vi "Unicorn.vi"() -> ()   [LabVIEW 2017, in "LV_Unicorn.lvlib"]
uses:
  LV_Unicorn.lvlib
  Control/AnswerUDP.ctl
  Control/unicorn_Param.ctl
  Control/unicorn_conn.ctl
  Control/unicorn_JSON.ctl
  Control/unicorn_ParamInt.ctl
  Control/unicorn_Telemetry.ctl
  Control/unicorn_Table.ctl
  Control/unicorn_ParamFloat.ctl
  Control/unicorn_array.ctl
  <vilib>/JDP Science/JSONtext/JSONtext.lvlib
panel:
  in  "FindMultiCast":bool
  in  "B_Connect":bool
  out "error out":errorcluster
  out "Ответ":string
  in  "B_Stop":bool
  in  "B_Disconnect":bool
  in  "Tab Control":T1(tab)=enum."Int"
  out "tblT":string[][](table) caption="Найденные устройства"
  in  "VersionControl":bool
  out "selDevices":T2
  in  "type_version":u32 format="%08x"
  out "devT":T2[](array[typedef])
  out "Cancel":bool
  out "ArrayUnicorn":T3
  in  "paramUnicorn":T4={"conParam"={"ReadIntParam"=TRUE, "ReadDescrParam"=FALSE, "ReadFloatParam"=TRUE, "debug"=FALSE, "ReadJSON"=TRUE, "IP_address"="192.168.1.227", "N_attempts"=5, "type_con"=enum."TCP", "MB_address"=1, "VISA"="COM1", "connection ID"=refnum, "nameDevices"="?`ОЦв-12, buld id Sep 17 2024 15:23:59", "timeout"=1000, "port"=2001, "type_version"="0A030001", "baud_rate"=115200, "VersionControl"=TRUE, "TCP_conn"=TRUE, "WindowSize"=700}, "Param"={"NumParam"={"NTelem"=201, "NInt"=16, "NFloat"=10, "NTable"=2}, "ParamInt"=[{"ID"="Режим работы", "Num"=0, "Name"="", "Type"="", "Enum"="", "Desc"="", "Unit"="", "Access"="", "FormatStr"="", "Min"=0, "Max"=0}, {"ID"="", "Num"=0, "Name"="", "Type"="", "Enum"="", "Desc"="", "Unit"="", "Access"="", "FormatStr"="", "Min"=0, "Max"=0}, {"ID"="", "Num"=0, "Name"="", "Type"="", "Enum"="", "Desc"="", "Unit"="", "Access"="", "FormatStr"="", "Min"=0, "Max"=0}, {"ID"="", "Num"=0, "Name"="", "Type"="", "Enum"="", "Desc"="", "Unit"="", "Access"="", "FormatStr"="", "Min"=0, "Max"=0}, {"ID"="", "Num"=0, "Name"="", "Type"="", "Enum"="", "Desc"="", "Unit"="", "Access"="", "FormatStr"="", "Min"=0, "Max"=0}, {"ID"="", "Num"=0, "Name"="", "Type"="", "Enum"="", "Desc"="", "Unit"="", "Access"="", "FormatStr"="", "Min"=0, "Max"=0}, {"ID"="ModeWork", "Num"=0, "Name"="", "Type"="", "Enum"="", "Desc"="", "Unit"="", "Access"="", "FormatStr"="", "Min"=0, "Max"=0}], "Telemetry"=[], "Table"=[], "ParamFloat"=[]}}
  in  "Pretty print":bool=TRUE
  out "JSONStr":string="{ \"UUID\": true, \"Reset\": false, \"Enums\": [ { \"ID\": \"Enum_LPF\", \"Name\": \"ФНЧ приемников\", \"Desc\": \"Частота среза фильтров низких частот\", \"Values\": [ { \"Name\": \"100\", \"Value\": 0, \"Desc\": \"\" }, { \"Name\": \"140\", \"Value\": 1, \"Desc\": \"\" } ] }, { \"ID\": \"Enum_HPF\", \"Name\": \"ФВЧ приемников\", \"Desc\": \"Частота среза фильтров высоких частот\", \"Values\": [ { \"Name\": \"5\", \"Value\": 0, \"Desc\": \"\" }, { \"Name\": \"10\", \"Value\": 1, \"Desc\": \"\" }, { \"Name\": \"20\", \"Value\": 2, \"Desc\": \"\" }, { \"Name\": \"40\", \"Value\": 3, \"Desc\": \"\" } ] }, { \"ID\": \"OnOffEnum\", \"Name\": \"On-off enum\", \"Num\": 0, \"Values\": [ { \"Name\": \"Выключено\", \"Value\": 0 }, { \"Name\": \"Включено\", \"Value\": 1 } ] } ], \"ParamInt\": [ { \"ID\": \"IPModeWork\", \"Num\": 0, \"Name\": \"Режим сканирования\", \"Type\": \"enum\", \"Enum\": \"OnOffEnum\", \"Desc\": \"Включение режима выполнения циклов сканирования\", \"Unit\": \"\", \"Access\": \"ro\" }, { \"ID\": \"IPStatusLF_EU\", \"Num\": 1, \"Name\": \"Состояние ЭБ НЧ\", \"Type\": \"Regular\", \"Desc\": \"Наличие ошибок в работе функциональных узлов ЭБ НЧ, при не нулевом значении светодиод «Состояние» мигает желтым или красным цветом\", \"Min\": 0, \"Max\": 0, \"Unit\": \"\", \"FormatStr\": \"0x%08x\", \"Access\": \"ro\" }, { \"ID\": \"IPGenNumber\", \"Num\": 2, \"Name\": \"Номер датчика для возбуждения\", \"Type\": \"Regular\", \"Desc\": \"Номер генератора который будет осуществлять возбуждение УЗ колебаний в ОК при помощи ПЭП, значение 0 отключает все генераторы\", \"Min\": 0, \"Max\": 16, \"Unit\": \"\", \"FormatStr\": \"%d\", \"Access\": \"rw\" }, { \"ID\": \"IPNumOfAvg\", \"Num\": 3, \"Name\": \"Количество усреднений принятых эхосигналов\", \"Type\": \"Regular\", \"Desc\": \"Количество повторений зондирования для усреднения принятых сигналов с ПЭП\", \"Min\": 1, \"Max\": 1023, \"Unit\": \"\", \"FormatStr\": \"%d\", \"Access\": \"rw\" }, { \"ID\": \"IPLPFilter\", \"Num\": 4, \"Name\": \"ФНЧ приемников\", \"Type\": \"enum\", \"Enum\": \"Enum_LPF\", \"Desc\": \"Частота среза фильтров низких частот приемников сигналов ПЭП\", \"Unit\": \"кГц\", \"Access\": \"rw\" }, { \"ID\": \"IPHPFilter\", \"Num\": 5, \"Name\": \"ФВЧ приемников\", \"Type\": \"enum\", \"Enum\": \"Enum_HPF\", \"Desc\": \"Частота среза фильтров высоких частот приемников сигналов ПЭП\", \"Unit\": \"кГц\", \"Access\": \"rw\" }, { \"ID\": \"IPModeTGC\", \"Num\": 6, \"Name\": \"Режим работы узла ВРЧ\", \"Desc\": \"Выбор режима работы узла управления временной регулировкой чувствительности\", \"Type\": \"enum\", \"Unit\": \"\", \"Access\": \"rw\", \"Enum\": { \"ID\": \"ModeTGCEnum\", \"Values\": [ { \"Desc\": \"В режиме «статический» используется не зависящая от времени чувствительность приемника\", \"Name\": \"Статический\", \"Value\": 0 }, { \"Desc\": \"В режиме «линейный» задается наклон изменения чувствительности в дБ/мс\", \"Name\": \"Линейный\", \"Value\": 1 }, { \"Desc\": \"В режиме «по таблице» значение чувствительности изменяется в соответствии с законом заданном в табличном виде\", \"Name\": \"По таблице\", \"Value\": 2 } ] } }, { \"ID\": \"IPFPGATypeVer\", \"Num\": 7, \"Name\": \"Тип и версия ПЛИС\", \"Type\": \"Regular\", \"Desc\": \"Тип и версия встроенного ПО ПЛИС платы АЦП ЭБ НЧ\", \"Unit\": \"\", \"FormatStr\": \"0x%08x\", \"Access\": \"ro\" }, { \"ID\": \"IPFPGABuildTime\", \"Num\": 8, \"Name\": \"Дата сборки ПО ПЛИС\", \"Type\": \"Regular\", \"Desc\": \"Дата сборки встроенного ПО ПЛИС платы АЦП\", \"Unit\": \"UNIX Time\", \"FormatStr\": \"%d\", \"Access\": \"ro\" }, { \"ID\": \"IPADCMonMCUBuildTime\", \"Num\": 9, \"Name\": \"Дата сборки ПО МК мониторинга платы АЦП\", \"Type\": \"Regular\", \"Desc\": \"Дата сборки ПО МК мониторинга платы АЦП\", \"Unit\": \"UNIX Time\", \"FormatStr\": \"%d\", \"Access\": \"ro\" }, { \"ID\": \"IPPMD2MCUBuildTime\", \"Num\": 10, \"Name\": \"Дата сборки ПО МК мониторинга ИП D2\", \"Type\": \"Regular\", \"Desc\": \"Дата сборки ПО МК мониторинга платы источника питания D2\", \"Unit\": \"UNIX Time\", \"FormatStr\": \"%d\", \"Access\": \"ro\" }, { \"ID\": \"IPPMD4MCUBuildTime\", \"Num\": 11, \"Name\": \"Дата сборки ПО МК мониторинга ИП D6\", \"Type\": \"Regular\", \"Desc\": \"Дата сборки ПО МК мониторинга платы источника питания D6\", \"Unit\": \"UNIX Time\", \"FormatStr\": \"%d\", \"Access\": \"ro\" }, { \"ID\": \"IPDefaultAddress\", \"Num\": 12, \"Name\": \"IP адрес электронного блока по умолчанию\", \"Type\": \"IPv4Addr\", \"Desc\": \"Присваивается электронному блоку если не был получен автоматически от DCHP сервера\", \"Unit\": \"IPv4\", \"Access\": \"rw\" }, { \"ID\": \"IPDefaultNetMask\", \"Num\": 13, \"Name\": \"Маска подсети\", \"Type\": \"IPv4Mask\", \"Desc\": \"Присваивается электронному блоку если не был получен автоматически от DCHP сервера\", \"Unit\": \"IPv4\", \"Access\": \"rw\" }, { \"ID\": \"IPDefaultGW\", \"Num\": 14, \"Name\": \"Основной шлюз \", \"Type\": \"IPv4Addr\", \"Desc\": \"Присваивается электронному блоку если не был получен автоматически от DCHP сервера\", \"Unit\": \"IPv4\", \"Access\": \"rw\" }, { \"ID\": \"IPSaveParem\", \"Num\": 15, \"Name\": \"Сохранение параметров\", \"Type\": \"bool\", \"Desc\": \"Сохранение параметров в энергонезависимую память\", \"Unit\": \"\", \"FormatStr\": \"\", \"Access\": \"rw\" } ], \"ParamFloat\": [ { \"ID\": \"FPFreqRepExPulses\", \"Num\": 0, \"Name\": \"Частота повторения импульсов возбуждения\", \"Desc\": \"Максимальная частота с которой будут формироваться импульсы возбуждения ПЭП\", \"Type\": \"Regular\", \"Unit\": \"Гц\", \"FormatStr\": \"%.1f\", \"Min\": 1.0, \"Max\": 20.0, \"Access\": \"rw\" }, { \"ID\": \"FPFreqExFilling\", \"Num\": 1, \"Name\": \"Частота сигнала заполнения импульса возбуждения\", \"Desc\": \"Частота сигнала заполнения импульса возбуждения ПЭП\", \"Type\": \"Regular\", \"Unit\": \"кГц\", \"FormatStr\": \"%.1f\", \"Min\": 10.0, \"Max\": 100.0, \"Access\": \"rw\" }, { \"ID\": \"FPNumPerFillExPulse\", \"Num\": 2, \"Name\": \"Количество периодов заполнения импульса возбуждения\", \"Desc\": \"Количество периодов частоты сигнала заполнения в импульсе возбуждения ПЭП\", \"Type\": \"Regular\", \"Unit\": \"шт\", \"FormatStr\": \"%.1f\", \"Min\": 1.0, \"Max\": 10.0, \"Access\": \"rw\" }, { \"ID\": \"FPAmplExPulse\", \"Num\": 3, \"Name\": \"Амплитуда импульса возбуждения\", \"Desc\": \"Максимальная амплитуда импульса возбуждения ПЭП, 100 % соответствуют 150 В амплитуды или 300 В размаха сигнала возбуждения ПЭП\", \"Type\": \"Regular\", \"Unit\": \"%\", \"FormatStr\": \"%.1f\", \"Min\": 0.0, \"Max\": 100.0, \"Access\": \"rw\" }, { \"ID\": \"FPDelayExPulse\", \"Num\": 4, \"Name\": \"Задержка начала импульса возбуждения\", \"Desc\": \"Задержка начала импульса возбуждения относительно импульса синхронизации\", \"Type\": \"Regular\", \"Unit\": \"мкс\", \"FormatStr\": \"%.2f\", \"Min\": 0.0, \"Max\": 50.0, \"Access\": \"rw\" }, { \"ID\": \"FPScanAreaDelay\", \"Num\": 5, \"Name\": \"Задержка области сканирования\", \"Desc\": \"Задержка начала области сканирования относительно импульса синхронизации, задержка начала работы приемников сигналов ПЭП\", \"Type\": \"Regular\", \"Unit\": \"мкс\", \"FormatStr\": \"%.2f\", \"Min\": 0.0, \"Max\": 100.0e3, \"Access\": \"rw\" }, { \"ID\": \"FPDurationScanArea\", \"Num\": 6, \"Name\": \"Длительность области сканирования\", \"Desc\": \"Длительность области сканирования, длительность работы приемников сигналов ПЭП\", \"Type\": \"Regular\", \"Unit\": \"мкс\", \"FormatStr\": \"%.2f\", \"Min\": 100.0, \"Max\": 15728.0, \"Access\": \"rw\" }, { \"ID\": \"FPSamplingFreq\", \"Num\": 7, \"Name\": \"Частота дискретизации сигнала принимаемого с ПЭП сигнала\", \"Desc\": \"Частота следования отсчетов амплитуды принятого с ПЭП эхосигнала\", \"Type\": \"Regular\", \"Unit\": \"Гц\", \"FormatStr\": \"%.2f\", \"Access\": \"ro\" }, { \"ID\": \"FPInitialGain\", \"Num\": 8, \"Name\": \"Начальное значение коэффициента усиления приемников\", \"Desc\": \"Значение усиления для режима работы ВРЧ «статический», для режимов «линейный» и «по таблице» используется как начальное значение усиления\", \"Type\": \"Regular\", \"Unit\": \"дБ\", \"FormatStr\": \"%.1f\", \"Min\": 0.0, \"Max\": 40.0, \"Access\": \"rw\" }, { \"ID\": \"FPRateChangeGain\", \"Num\": 9, \"Name\": \"Скорость изменения чувствительности\", \"Desc\": \"Значение скорости изменения усиления для режима работы ВРЧ «линейный», в режимах «статический» и «по таблице» не влияет на работу узла ВРЧ\", \"Type\": \"Regular\", \"Unit\": \"дБ/мс\", \"FormatStr\": \"%.2f\", \"Min\": -40.0, \"Max\": 40.0, \"Access\": \"rw\" } ], \"Telemetry\": [ { \"ID\": \"CoreUptime\", \"Num\": 0, \"Name\": \"Core uptime\", \"Desc\": \"\", \"Unit\": \"s\", \"FormatStr\": \"%.1f\" }, { \"ID\": \"LCUptime\", \"Num\": 1, \"Name\": \"FPGA uptime\", \"Desc\": \"\", \"Unit\": \"s\", \"FormatStr\": \"%.1f\" }, { \"ID\": \"TelStatusLF_EU\", \"Num\": 2, \"Name\": \"TelStatusLF_EU\", \"Desc\": \"\", \"Unit\": \"\", \"Min\": -0.01, \"Max\": 0.01, \"FormatStr\": \"%.0f\" }, { \"ID\": \"TelMBVrefMin\", \"Num\": 3, \"Name\": \"TelMBVrefMin\", \"Desc\": \"\", \"Unit\": \"В\", \"Min\": 1.18, \"Max\": 1.22, \"FormatStr\": \"%.3f\" }, { \"ID\": \"TelMBVrefAvg\", \"Num\": 4, \"Name\": \"TelMBVrefAvg\", \"Desc\": \"\", \"Unit\": \"В\", \"Min\": 1.18, \"Max\": 1.22, \"FormatStr\": \"%.3f\" }, { \"ID\": \"TelMBVrefMax\", \"Num\": 5, \"Name\": \"TelMBVrefMax\", \"Desc\": \"\", \"Unit\": \"В\", \"Min\": 1.18, \"Max\": 1.22, \"FormatStr\": \"%.3f\" }, { \"ID\": \"TelMB3_3VMin\", \"Num\": 6, \"Name\": \"TelMB3_3VMin\", \"Desc\": \"\", \"Unit\": \"В\", \"Min\": 3.2, \"Max\": 3.45, \"FormatStr\": \"%.3f\" }, { \"ID\": \"TelMB3_3VAvg\", \"Num\": 7, \"Name\": \"TelMB3_3VAvg\", \"Desc\": \"\", \"Unit\": \"В\", \"Min\": 3.2, \"Max\": 3.45, \"FormatStr\": \"%.3f\" }, { \"ID\": \"TelMB3_3VMax\", \"Num\": 8, \"Name\": \"TelMB3_3VMax\", \"Desc\": \"\", \"Unit\": \"В\", \"Min\": 3.2, \"Max\": 3.45, \"FormatStr\": \"%.3f\" }, { \"ID\": \"TelMB3_3VcMin\", \"Num\": 9, \"Name\": \"TelMB3_3VcMin\", \"Desc\": \"\", \"Unit\": \"В\", \"Min\": 3.2, \"Max\": 3.45, \"FormatStr\": \"%.3f\" }, { \"ID\": \"TelMB3_3VcAvg\", \"Num\": 10, \"Name\": \"TelMB3_3VcAvg\", \"Desc\": \"\", \"Unit\": \"В\", \"Min\": 3.2, \"Max\": 3.45, \"FormatStr\": \"%.3f\" }, { \"ID\": \"TelMB3_3VcMax\", \"Num\": 11, \"Name\": \"TelMB3_3VcMax\", \"Desc\": \"\", \"Unit\": \"В\", \"Min\": 3.2, \"Max\": 3.45, \"FormatStr\": \"%.3f\" }, { \"ID\": \"TelMB1_8VcMin\", \"Num\": 12, \"Name\": \"TelMB1_8VcMin\", \"Desc\": \"\", \"Unit\": \"В\", \"Min\": 1.65, \"Max\": 1.95, \"FormatStr\": \"%.3f\" }, { \"ID\": \"TelMB1_8VcAvg\", \"Num\": 13, \"Name\": \"TelMB1_8VcAvg\", \"Desc\": \"\", \"Unit\": \"В\", \"Min\": 1.65, \"Max\": 1.95, \"FormatStr\": \"%.3f\" }, { \"ID\": \"TelMB1_8VcMax\", \"Num\": 14, \"Name\": \"TelMB1_8VcMax\", \"Desc\": \"\", \"Unit\": \"В\", \"Min\": 1.65, \"Max\": 1.95, \"FormatStr\": \"%.3f\" }, { \"ID\": \"TelMB5VcMin\", \"Num\": 15, \"Name\": \"TelMB5VcMin\", \"Desc\": \"\", \"Unit\": \"В\", \"Min\": 4.8, \"Max\": 5.25, \"FormatStr\": \"%.3f\" }, { \"ID\": \"TelMB5VcAvg\", \"Num\": 16, \"Name\": \"TelMB5VcAvg\", \"Desc\": \"\", \"Unit\": \"В\", \"Min\": 4.8, \"Max\": 5.25, \"FormatStr\": \"%.3f\" }, { \"ID\": \"TelMB5VcMax\", \"Num\": 17, \"Name\": \"TelMB5VcMax\", \"Desc\": \"\", \"Unit\": \"В\", \"Min\": 4.8, \"Max\": 5.25, \"FormatStr\": \"%.3f\" }, { \"ID\": \"TelMB5VconMin\", \"Num\": 18, \"Name\": \"TelMB5VconMin\", \"Desc\": \"\", \"Unit\": \"В\", \"Min\": 4.8, \"Max\": 5.25, \"FormatStr\": \"%.3f\" }, { \"ID\": \"TelMB5VconAvg\", \"Num\": 19, \"Name\": \"TelMB5VconAvg\", \"Desc\": \"\", \"Unit\": \"В\", \"Min\": 4.8, \"Max\": 5.25, \"FormatStr\": \"%.3f\" }, { \"ID\": \"_TelMB5VconMax\", \"Num\": 20, \"Name\": \"_TelMB5VconMax\", \"Desc\": \"\", \"Unit\": \"В\", \"Min\": 4.8, \"Max\": 5.25, \"FormatStr\": \"%.3f\" }, { \"ID\": \"TelMBTemp\", \"Num\": 21, \"Name\": \"TelMBTemp\", \"Desc\": \"\", \"Unit\": \"°C\", \"Min\": 10.0, \"Max\": 80.0, \"FormatStr\": \"%.1f\" }, { \"ID\": \"TelADCGDUptime\", \"Num\": 22, \"Name\": \"TelADCGDUptime\", \"Desc\": \"\", \"Unit\": \"s\", \"FormatStr\": \"%.0f\" }, { \"ID\": \"TelADCVRefIntMin\", \"Num\": 23, \"Name\": \"TelADCVRefIntMin\", \"Desc\": \"\", \"Unit\": \"V\", \"Min\": 1.18, \"Max\": 1.22, \"FormatStr\": \"%.3f\" }, { \"ID\": \"TelADCVRefIntAVG\", \"Num\": 24, \"Name\": \"TelADCVRefIntAVG\", \"Desc\": \"\", \"Unit\": \"V\", \"Min\": 1.18, \"Max\": 1.22, \"FormatStr\": \"%.3f\" }, { \"ID\": \"TelADCVRefIntMax\", \"Num\": 25, \"Name\": \"TelADCVRefIntMax\", \"Desc\": \"\", \"Unit\": \"V\", \"Min\": 1.18, \"Max\": 1.22, \"FormatStr\": \"%.3f\" }, { \"ID\": \"TelADCVp1_2VdMin\", \"Num\": 26, \"Name\": \"TelADCVp1_2VdMin\", \"Desc\": \"\", \"Unit\": \"V\", \"Min\": 1.18, \"Max\": 1.28, \"FormatStr\": \"%.3f\" }, { \"ID\": \"TelADCVp1_2VdAVG\", \"Num\": 27, \"Name\": \"TelADCVp1_2VdAVG\", \"Desc\": \"\", \"Unit\": \"V\", \"Min\": 1.18, \"Max\": 1.28, \"FormatStr\": \"%.3f\" }, { \"ID\": \"TelADCVp1_2VdMax\", \"Num\": 28, \"Name\": \"TelADCVp1_2VdMax\", \"Desc\": \"\", \"Unit\": \"V\", \"Min\": 1.18, \"Max\": 1.28, \"FormatStr\": \"%.3f\" }, { \"ID\": \"TelADCVp1_8VaMin\", \"Num\": 29, \"Name\": \"TelADCVp1_8VaMin\", \"Desc\": \"\", \"Unit\": \"V\", \"Min\": 1.65, \"Max\": 1.95, \"FormatStr\": \"%.3f\" }, { \"ID\": \"TelADCVp1_8VaAVG\", \"Num\": 30, \"Name\": \"TelADCVp1_8VaAVG\", \"Desc\": \"\", \"Unit\": \"V\", \"Min\": 1.65, \"Max\": 1.95, \"FormatStr\": \"%.3f\" }, { \"ID\": \"TelADCVp1_8VaMax\", \"Num\": 31, \"Name\": \"TelADCVp1_8VaMax\", \"Desc\": \"\", \"Unit\": \"V\", \"Min\": 1.65, \"Max\": 1.95, \"FormatStr\": \"%.3f\" }, { \"ID\": \"TelADCVp3_3VMin\", \"Num\": 32, \"Name\": \"TelADCVp3_3VMin\", \"Desc\": \"\", \"Unit\": \"V\", \"Min\": 3.2, \"Max\": 3.45, \"FormatStr\": \"%.3f\" }, { \"ID\": \"TelADCVp3_3VAVG\", \"Num\": 33, \"Name\": \"TelADCVp3_3VAVG\", \"Desc\": \"\", \"Unit\": \"V\", \"Min\": 3.2, \"Max\": 3.45, \"FormatStr\": \"%.3f\" }, { \"ID\": \"TelADCVp3_3VMax\", \"Num\": 34, \"Name\": \"TelADCVp3_3VMax\", \"Desc\": \"\", \"Unit\": \"V\", \"Min\": 3.2, \"Max\": 3.45, \"FormatStr\": \"%.3f\" }, { \"ID\": \"TelADCVp5VMin\", \"Num\": 35, \"Name\": \"TelADCVp5VMin\", \"Desc\": \"\", \"Unit\": \"V\", \"Min\": 4.8, \"Max\": 5.25, \"FormatStr\": \"%.3f\" }, { \"ID\": \"TelADCVp5VAVG\", \"Num\": 36, \"Name\": \"TelADCVp5VAVG\", \"Desc\": \"\", \"Unit\": \"V\", \"Min\": 4.8, \"Max\": 5.25, \"FormatStr\": \"%.3f\" }, { \"ID\": \"TelADCVp5VMax\", \"Num\": 37, \"Name\": \"TelADCVp5VMax\", \"Desc\": \"\", \"Unit\": \"V\", \"Min\": 4.8, \"Max\": 5.25, \"FormatStr\": \"%.3f\" }, { \"ID\": \"TelADCVp5VsMin\", \"Num\": 38, \"Name\": \"TelADCVp5VsMin\", \"Desc\": \"\", \"Unit\": \"V\", \"Min\": 4.8, \"Max\": 5.25, \"FormatStr\": \"%.3f\" }, { \"ID\": \"TelADCVp5VsAVG\", \"Num\": 39, \"Name\": \"TelADCVp5VsAVG\", \"Desc\": \"\", \"Unit\": \"V\", \"Min\": 4.8, \"Max\": 5.25, \"FormatStr\": \"%.3f\" }, { \"ID\": \"TelADCVp5VsMax\", \"Num\": 40, \"Name\": \"TelADCVp5VsMax\", \"Desc\": \"\", \"Unit\": \"V\", \"Min\": 4.8, \"Max\": 5.25, \"FormatStr\": \"%.3f\" }, { \"ID\": \"TelADCVp15VMin\", \"Num\": 41, \"Name\": \"TelADCVp15VMin\", \"Desc\": \"\", \"Unit\": \"V\", \"Min\": 14.5, \"Max\": 15.5, \"FormatStr\": \"%.3f\" }, { \"ID\": \"TelADCVp15VAVG\", \"Num\": 42, \"Name\": \"TelADCVp15VAVG\", \"Desc\": \"\", \"Unit\": \"V\", \"Min\": 14.5, \"Max\": 15.5, \"FormatStr\": \"%.3f\" }, { \"ID\": \"TelADCVp15VMax\", \"Num\": 43, \"Name\": \"TelADCVp15VMax\", \"Desc\": \"\", \"Unit\": \"V\", \"Min\": 14.5, \"Max\": 15.5, \"FormatStr\": \"%.3f\" }, { \"ID\": \"TelADCVn5VMin\", \"Num\": 44, \"Name\": \"TelADCVn5VMin\", \"Desc\": \"\", \"Unit\": \"V\", \"Min\": -5.25, \"Max\": -4.8, \"FormatStr\": \"%.3f\" }, { \"ID\": \"TelADCVn5VAVG\", \"Num\": 45, \"Name\": \"TelADCVn5VAVG\", \"Desc\": \"\", \"Unit\": \"V\", \"Min\": -5.25, \"Max\": -4.8, \"FormatStr\": \"%.3f\" }, { \"ID\": \"TelADCVn5VMax\", \"Num\": 46, \"Name\": \"TelADCVn5VMax\", \"Desc\": \"\", \"Unit\": \"V\", \"Min\": -5.25, \"Max\": -4.8, \"FormatStr\": \"%.3f\" }, { \"ID\": \"TelADCVn15VMin\", \"Num\": 47, \"Name\": \"TelADCVn15VMin\", \"Desc\": \"\", \"Unit\": \"V\", \"Min\": -15.5, \"Max\": -14.5, \"FormatStr\": \"%.3f\" }, { \"ID\": \"TelADCVn15VAVG\", \"Num\": 48, \"Name\": \"TelADCVn15VAVG\", \"Desc\": \"\", \"Unit\": \"V\", \"Min\": -15.5, \"Max\": -14.5, \"FormatStr\": \"%.3f\" }, { \"ID\": \"TelADCVn15VMax\", \"Num\": 49, \"Name\": \"TelADCVn15VMax\", \"Desc\": \"\", \"Unit\": \"V\", \"Min\": -15.5, \"Max\": -14.5, \"FormatStr\": \"%.3f\" }, { \"ID\": \"TelADCTempSensor\", \"Num\": 50, \"Name\": \"TelADCTempSensor\", \"Desc\": \"\", \"Unit\": \"°C\", \"Min\": 10.0, \"Max\": 80.0, \"FormatStr\": \"%.1f\" }, { \"ID\": \"TelGD32E230PassPacketCount\", \"Num\": 51, \"Name\": \"TelGD32E230PassPacketCount\", \"Desc\": \"\", \"Unit\": \"\", \"FormatStr\": \"%.0f\" }, { \"ID\": \"TelGD32E230ErrorPacketCount\", \"Num\": 52, \"Name\": \"TelGD32E230ErrorPacketCount\", \"Desc\": \"\", \"Unit\": \"\", \"FormatStr\": \"%.0f\" }, { \"ID\": \"TelPMD2Up_time\", \"Num\": 53, \"Name\": \"PM D2 Uptime\", \"Desc\": \"\", \"Unit\": \"s\", \"FormatStr\": \"%.0f\" }, { \"ID\": \"TelPMD2CInMin\", \"Num\": 54, \"Name\": \"TelPMD2CInMin\", \"Desc\": \"\", \"Unit\": \"A\", \"Min\": 0.1, \"Max\": 3.15, \"FormatStr\": \"%.3f\" }, { \"ID\": \"TelPMD2CInAVG\", \"Num\": 55, \"Name\": \"TelPMD2CInAVG\", \"Desc\": \"\", \"Unit\": \"A\", \"Min\": 0.1, \"Max\": 3.15, \"FormatStr\": \"%.3f\" }, { \"ID\": \"TelPMD2CInMax\", \"Num\": 56, \"Name\": \"TelPMD2CInMax\", \"Desc\": \"\", \"Unit\": \"A\", \"Min\": 0.1, \"Max\": 3.15, \"FormatStr\": \"%.3f\" }, { \"ID\": \"TelPMD2VInMin\", \"Num\": 57, \"Name\": \"TelPMD2VInMin\", \"Desc\": \"\", \"Unit\": \"V\", \"Min\": 10.5, \"Max\": 14.0, \"FormatStr\": \"%.3f\" }, { \"ID\": \"TelPMD2VInAVG\", \"Num\": 58, \"Name\": \"TelPMD2VInAVG\", \"Desc\": \"\", \"Unit\": \"V\", \"Min\": 10.5, \"Max\": 14.0, \"FormatStr\": \"%.3f\" }, { \"ID\": \"TelPMD2VInMax\", \"Num\": 59, \"Name\": \"TelPMD2VInMax\", \"Desc\": \"\", \"Unit\": \"V\", \"Min\": 10.5, \"Max\": 14.0, \"FormatStr\": \"%.3f\" }, { \"ID\": \"TelPMD2PInMin\", \"Num\": 60, \"Name\": \"TelPMD2PInMin\", \"Desc\": \"\", \"Unit\": \"W\", \"Min\": 1.0, \"Max\": 30.0, \"FormatStr\": \"%.3f\" }, { \"ID\": \"TelPMD2PInAVG\", \"Num\": 61, \"Name\": \"TelPMD2PInAVG\", \"Desc\": \"\", \"Unit\": \"W\", \"Min\": 1.0, \"Max\": 30.0, \"FormatStr\": \"%.3f\" }, { \"ID\": \"TelPMD2PInMax\", \"Num\": 62, \"Name\": \"TelPMD2PInMax\", \"Desc\": \"\", \"Unit\": \"W\", \"Min\": 1.0, \"Max\": 30.0, \"FormatStr\": \"%.3f\" }, { \"ID\": \"TelPMD2VRefIntMin\", \"Num\": 63, \"Name\": \"TelPMD2VRefIntMin\", \"Desc\": \"\", \"Unit\": \"V\", \"Min\": 1.18, \"Max\": 1.22, \"FormatStr\": \"%.3f\" }, { \"ID\": \"TelPMD2VRefIntAVG\", \"Num\": 64, \"Name\": \"TelPMD2VRefIntAVG\", \"Desc\": \"\", \"Unit\": \"V\", \"Min\": 1.18, \"Max\": 1.22, \"FormatStr\": \"%.3f\" }, { \"ID\": \"TelPMD2VRefIntMax\", \"Num\": 65, \"Name\": \"TelPMD2VRefIntMax\", \"Desc\": \"\", \"Unit\": \"V\", \"Min\": 1.18, \"Max\": 1.22, \"FormatStr\": \"%.3f\" }, { \"ID\": \"TelPMD2ConvFreq\", \"Num\": 66, \"Name\": \"TelPMD2ConvFreq\", \"Desc\": \"\", \"Unit\": \"Hz\", \"Min\": 120.0e3, \"Max\": 135.0e3, \"FormatStr\": \"%.0f\" }, { \"ID\": \"TelPMD2TempSensor\", \"Num\": 67, \"Name\": \"TelPMD2TempSensor\", \"Desc\": \"\", \"Unit\": \"°C\", \"Min\": 10.0, \"Max\": 80.0, \"FormatStr\": \"%.1f\" }, { \"ID\": \"TelPMD6Up_time\", \"Num\": 68, \"Name\": \"PM D6 Uptime\", \"Desc\": \"\", \"Unit\": \"s\", \"FormatStr\": \"%.0f\" }, { \"ID\": \"TelPMD6Vp45VMin\", \"Num\": 69, \"Name\": \"TelPMD6Vp45VMin\", \"Desc\": \"\", \"Unit\": \"V\", \"Min\": 42.0, \"Max\": 47.0, \"FormatStr\": \"%.3f\" }, { \"ID\": \"TelPMD6Vp45VAVG\", \"Num\": 70, \"Name\": \"TelPMD6Vp45VAVG\", \"Desc\": \"\", \"Unit\": \"V\", \"Min\": 42.0, \"Max\": 47.0, \"FormatStr\": \"%.3f\" }, { \"ID\": \"TelPMD6Vp45VMax\", \"Num\": 71, \"Name\": \"TelPMD6Vp45VMax\", \"Desc\": \"\", \"Unit\": \"V\", \"Min\": 42.0, \"Max\": 47.0, \"FormatStr\": \"%.3f\" }, { \"ID\": \"TelPMD6Vn45VMin\", \"Num\": 72, \"Name\": \"TelPMD6Vn45VMin\", \"Desc\": \"\", \"Unit\": \"V\", \"Min\": -47.0, \"Max\": -42.0, \"FormatStr\": \"%.3f\" }, { \"ID\": \"TelPMD6Vn45VAVG\", \"Num\": 73, \"Name\": \"TelPMD6Vn45VAVG\", \"Desc\": \"\", \"Unit\": \"V\", \"Min\": -47.0, \"Max\": -42.0, \"FormatStr\": \"%.3f\" }, { \"ID\": \"TelPMD6Vn45VMax\", \"Num\": 74, \"Name\": \"TelPMD6Vn45VMax\", \"Desc\": \"\", \"Unit\": \"V\", \"Min\": -47.0, \"Max\": -42.0, \"FormatStr\": \"%.3f\" }, { \"ID\": \"TelPMD6Vp8VMin\", \"Num\": 75, \"Name\": \"TelPMD6Vp8VMin\", \"Desc\": \"\", \"Unit\": \"V\", \"Min\": 7.0, \"Max\": 9.5, \"FormatStr\": \"%.3f\" }, { \"ID\": \"TelPMD6Vp8VAVG\", \"Num\": 76, \"Name\": \"TelPMD6Vp8VAVG\", \"Desc\": \"\", \"Unit\": \"V\", \"Min\": 7.0, \"Max\": 9.5, \"FormatStr\": \"%.3f\" }, { \"ID\": \"TelPMD6Vp8VMax\", \"Num\": 77, \"Name\": \"TelPMD6Vp8VMax\", \"Desc\": \"\", \"Unit\": \"V\", \"Min\": 7.0, \"Max\": 9.5, \"FormatStr\": \"%.3f\" }, { \"ID\": \"TelPMD6Vp5VMin\", \"Num\": 78, \"Name\": \"TelPMD6Vp5VMin\", \"Desc\": \"\", \"Unit\": \"V\", \"Min\": 4.8, \"Max\": 5.3, \"FormatStr\": \"%.3f\" }, { \"ID\": \"TelPMD6Vp5VAVG\", \"Num\": 79, \"Name\": \"TelPMD6Vp5VAVG\", \"Desc\": \"\", \"Unit\": \"V\", \"Min\": 4.8, \"Max\": 5.3, \"FormatStr\": \"%.3f\" }, { \"ID\": \"TelPMD6Vp5VMax\", \"Num\": 80, \"Name\": \"TelPMD6Vp5VMax\", \"Desc\": \"\", \"Unit\": \"V\", \"Min\": 4.8, \"Max\": 5.3, \"FormatStr\": \"%.3f\" }, { \"ID\": \"TelPMD6Vp20VMin\", \"Num\": 81, \"Name\": \"TelPMD6Vp20VMin\", \"Desc\": \"\", \"Unit\": \"V\", \"Min\": 17.0, \"Max\": 19.0, \"FormatStr\": \"%.3f\" }, { \"ID\": \"TelPMD6Vp20VAVG\", \"Num\": 82, \"Name\": \"TelPMD6Vp20VAVG\", \"Desc\": \"\", \"Unit\": \"V\", \"Min\": 17.0, \"Max\": 19.0, \"FormatStr\": \"%.3f\" }, { \"ID\": \"TelPMD6Vp20VMax\", \"Num\": 83, \"Name\": \"TelPMD6Vp20VMax\", \"Desc\": \"\", \"Unit\": \"V\", \"Min\": 17.0, \"Max\": 19.0, \"FormatStr\": \"%.3f\" }, { \"ID\": \"TelPMD6Vn8VMin\", \"Num\": 84, \"Name\": \"TelPMD6Vn8VMin\", \"Desc\": \"\", \"Unit\": \"V\", \"Min\": -9.5, \"Max\": -7.0, \"FormatStr\": \"%.3f\" }, { \"ID\": \"TelPMD6Vn8VAVG\", \"Num\": 85, \"Name\": \"TelPMD6Vn8VAVG\", \"Desc\": \"\", \"Unit\": \"V\", \"Min\": -9.5, \"Max\": -7.0, \"FormatStr\": \"%.3f\" }, { \"ID\": \"TelPMD6Vn8VMax\", \"Num\": 86, \"Name\": \"TelPMD6Vn8VMax\", \"Desc\": \"\", \"Unit\": \"V\", \"Min\": -9.5, \"Max\": -7.0, \"FormatStr\": \"%.3f\" }, { \"ID\": \"TelPMD6Vn20VMin\", \"Num\": 87, \"Name\": \"TelPMD6Vn20VMin\", \"Desc\": \"\", \"Unit\": \"V\", \"Min\": -19.0, \"Max\": -17.0, \"FormatStr\": \"%.3f\" }, { \"ID\": \"TelPMD6Vn20VAVG\", \"Num\": 88, \"Name\": \"TelPMD6Vn20VAVG\", \"Desc\": \"\", \"Unit\": \"V\", \"Min\": -19.0, \"Max\": -17.0, \"FormatStr\": \"%.3f\" }, { \"ID\": \"TelPMD6Vn20VMax\", \"Num\": 89, \"Name\": \"TelPMD6Vn20VMax\", \"Desc\": \"\", \"Unit\": \"V\", \"Min\": -19.0, \"Max\": -17.0, \"FormatStr\": \"%.3f\" }, { \"ID\": \"TelPMD6VRefIntMin\", \"Num\": 90, \"Name\": \"TelPMD6VRefIntMin\", \"Desc\": \"\", \"Unit\": \"V\", \"Min\": 1.18, \"Max\": 1.22, \"FormatStr\": \"%.3f\" }, { \"ID\": \"TelPMD6VRefIntAVG\", \"Num\": 91, \"Name\": \"TelPMD6VRefIntAVG\", \"Desc\": \"\", \"Unit\": \"V\", \"Min\": 1.18, \"Max\": 1.22, \"FormatStr\": \"%.3f\" }, { \"ID\": \"TelPMD6VRefIntMax\", \"Num\": 92, \"Name\": \"TelPMD6VRefIntMax\", \"Desc\": \"\", \"Unit\": \"V\", \"Min\": 1.18, \"Max\": 1.22, \"FormatStr\": \"%.3f\" }, { \"ID\": \"TelPMD6TempSensor\", \"Num\": 93, \"Name\": \"TelPMD6TempSensor\", \"Desc\": \"\", \"Unit\": \"°C\", \"Min\": 10.0, \"Max\": 80.0, \"FormatStr\": \"%.1f\" }, { \"ID\": \"TelPMPassPacketCount\", \"Num\": 94, \"Name\": \"TelPMPassPacketCount\", \"Desc\": \"\", \"Unit\": \"\", \"FormatStr\": \"%.0f\" }, { \"ID\": \"TelPMErrorPacketCount\", \"Num\": 95, \"Name\": \"TelPMErrorPacketCount\", \"Desc\": \"\", \"Unit\": \"\", \"FormatStr\": \"%.0f\" } ], \"Table\": [ { \"Num\": 0, \"Access\": \"ro\", \"ColumnCount\": 18, \"DataType\": \"float\", \"FormatStr\": \"%f\", \"ID\": \"RAWADCData\", \"Name\": \"Данные АЦП\", \"NeedParamPrepare\": true, \"RowCount\": 1, \"Columns\": [ { \"Column\": 0, \"Name\": \"Ось времени\", \"Type\": \"Regular\" },{ \"Column\": 1, \"Name\": \"Датчик 1\", \"Type\": \"Regular\" },{ \"Column\": 2, \"Name\": \"Датчик 2\", \"Type\": \"Regular\" },{ \"Column\": 3, \"Name\": \"Датчик 3\", \"Type\": \"Regular\" },{ \"Column\": 4, \"Name\": \"Датчик 4\", \"Type\": \"Regular\" },{ \"Column\": 5, \"Name\": \"Датчик 5\", \"Type\": \"Regular\" },{ \"Column\": 6, \"Name\": \"Датчик 6\", \"Type\": \"Regular\" },{ \"Column\": 7, \"Name\": \"Датчик 7\", \"Type\": \"Regular\" },{ \"Column\": 8, \"Name\": \"Датчик 8\", \"Type\": \"Regular\" },{ \"Column\": 9, \"Name\": \"Датчик 9\", \"Type\": \"Regular\" },{ \"Column\": 10, \"Name\": \"Датчик 10\", \"Type\": \"Regular\" },{ \"Column\": 11, \"Name\": \"Датчик 11\", \"Type\": \"Regular\" },{ \"Column\": 12, \"Name\": \"Датчик 12\", \"Type\": \"Regular\" },{ \"Column\": 13, \"Name\": \"Датчик 13\", \"Type\": \"Regular\" },{ \"Column\": 14, \"Name\": \"Датчик 14\", \"Type\": \"Regular\" },{ \"Column\": 15, \"Name\": \"Датчик 15\", \"Type\": \"Regular\" },{ \"Column\": 16, \"Name\": \"Датчик 16\", \"Type\": \"Regular\" },{ \"Column\": 17, \"Name\": \"Коэфф. усиления\", \"Type\": \"Regular\" } ] }, { \"Num\": 1, \"ID\": \"CalibrADC\", \"Access\": \"rw\", \"ColumnCount\": 2, \"RowCount\": 16, \"DataType\": \"float\", \"FormatStr\": \"%f\", \"Name\": \"Параметры калибровки\", \"Desc\": \"Параметры калибровки каналов приема\", \"NeedParamPrepare\": false, \"Columns\": [ { \"Column\": 0, \"Name\": \"Смещение\", \"Type\": \"Regular\" },{ \"Column\": 1, \"Name\": \"Коэфф.\", \"Type\": \"Regular\" } ], \"Rows\": [ { \"Row\": 0, \"Name\": \"Канал 1\", \"Type\": \"Regular\" },{ \"Row\": 1, \"Name\": \"Канал 2\", \"Type\": \"Regular\" },{ \"Row\": 2, \"Name\": \"Канал 3\", \"Type\": \"Regular\" },{ \"Row\": 3, \"Name\": \"Канал 4\", \"Type\": \"Regular\" },{ \"Row\": 4, \"Name\": \"Канал 5\", \"Type\": \"Regular\" },{ \"Row\": 5, \"Name\": \"Канал 6\", \"Type\": \"Regular\" },{ \"Row\": 6, \"Name\": \"Канал 7\", \"Type\": \"Regular\" },{ \"Row\": 7, \"Name\": \"Канал 8\", \"Type\": \"Regular\" },{ \"Row\": 8, \"Name\": \"Канал 9\", \"Type\": \"Regular\" },{ \"Row\": 9, \"Name\": \"Канал 10\", \"Type\": \"Regular\" },{ \"Row\": 10, \"Name\": \"Канал 11\", \"Type\": \"Regular\" },{ \"Row\": 11, \"Name\": \"Канал 12\", \"Type\": \"Regular\" },{ \"Row\": 12, \"Name\": \"Канал 13\", \"Type\": \"Regular\" },{ \"Row\": 13, \"Name\": \"Канал 14\", \"Type\": \"Regular\" },{ \"Row\": 14, \"Name\": \"Канал 15\", \"Type\": \"Regular\" },{ \"Row\": 15, \"Name\": \"Канал 16\", \"Type\": \"Regular\" } ] } ] }"
  in  "ReadJSON":bool
  in  "ReadOneTelem":bool
  out "TableTelem":string[][](table)=[["1", "Core uptime", "13651.2", "s"], ["2", "FPGA uptime", "13651.2", "s"], ["3", "TelStatusLF_EU", "0", ""], ["4", "TelMBVrefMin", "1.188", "В"], ["5", "TelMBVrefAvg", "1.195", "В"], ["6", "TelMBVrefMax", "1.200", "В"], ["7", "TelMB3_3VMin", "3.284", "В"], ["8", "TelMB3_3VAvg", "3.293", "В"], ["9", "TelMB3_3VMax", "3.300", "В"], ["10", "TelMB3_3VcMin", "3.284", "В"], ["11", "TelMB3_3VcAvg", "3.291", "В"], ["12", "TelMB3_3VcMax", "3.297", "В"], ["13", "TelMB1_8VcMin", "1.826", "В"], ["14", "TelMB1_8VcAvg", "1.831", "В"], ["15", "TelMB1_8VcMax", "1.836", "В"], ["16", "TelMB5VcMin", "4.919", "В"], ["17", "TelMB5VcAvg", "4.932", "В"], ["18", "TelMB5VcMax", "4.943", "В"], ["19", "TelMB5VconMin", "4.951", "В"], ["20", "TelMB5VconAvg", "4.978", "В"], ["21", "_TelMB5VconMax", "4.995", "В"], ["22", "TelMBTemp", "58.1", "°C"], ["23", "TelADCGDUptime", "13682", "s"], ["24", "TelADCVRefIntMin", "1.197", "V"], ["25", "TelADCVRefIntAVG", "1.200", "V"], ["26", "TelADCVRefIntMax", "1.203", "V"], ["27", "TelADCVp1_2VdMin", "1.280", "V"], ["28", "TelADCVp1_2VdAVG", "1.284", "V"], ["29", "TelADCVp1_2VdMax", "1.287", "V"], ["30", "TelADCVp1_8VaMin", "1.873", "V"], ["31", "TelADCVp1_8VaAVG", "1.879", "V"], ["32", "TelADCVp1_8VaMax", "1.885", "V"], ["33", "TelADCVp3_3VMin", "3.401", "V"], ["34", "TelADCVp3_3VAVG", "3.402", "V"], ["35", "TelADCVp3_3VMax", "3.410", "V"], ["36", "TelADCVp5VMin", "5.148", "V"], ["37", "TelADCVp5VAVG", "5.170", "V"], ["38", "TelADCVp5VMax", "5.192", "V"], ["39", "TelADCVp5VsMin", "5.082", "V"], ["40", "TelADCVp5VsAVG", "5.090", "V"], ["41", "TelADCVp5VsMax", "5.098", "V"], ["42", "TelADCVp15VMin", "15.311", "V"], ["43", "TelADCVp15VAVG", "15.392", "V"], ["44", "TelADCVp15VMax", "15.453", "V"], ["45", "TelADCVn5VMin", "-5.170", "V"], ["46", "TelADCVn5VAVG", "-5.153", "V"], ["47", "TelADCVn5VMax", "-5.132", "V"], ["48", "TelADCVn15VMin", "-15.523", "V"], ["49", "TelADCVn15VAVG", "-15.457", "V"], ["50", "TelADCVn15VMax", "-15.390", "V"], ["51", "TelADCTempSensor", "44.1", "°C"], ["52", "TelGD32E230PassPacketCount", "13547", ""], ["53", "TelGD32E230ErrorPacketCount", "1", ""], ["54", "PM D2 Uptime", "13607", "s"], ["55", "TelPMD2CInMin", "3.500", "A"], ["56", "TelPMD2CInAVG", "3.588", "A"], ["57", "TelPMD2CInMax", "3.700", "A"], ["58", "TelPMD2VInMin", "10.708", "V"], ["59", "TelPMD2VInAVG", "10.790", "V"], ["60", "TelPMD2VInMax", "10.866", "V"], ["61", "TelPMD2PInMin", "37.045", "W"], ["62", "TelPMD2PInAVG", "37.871", "W"], ["63", "TelPMD2PInMax", "38.917", "W"], ["64", "TelPMD2VRefIntMin", "1.198", "V"], ["65", "TelPMD2VRefIntAVG", "1.201", "V"], ["66", "TelPMD2VRefIntMax", "1.204", "V"], ["67", "TelPMD2ConvFreq", "116865", "Hz"], ["68", "TelPMD2TempSensor", "69.2", "°C"], ["69", "PM D6 Uptime", "13686", "s"], ["70", "TelPMD6Vp45VMin", "32.202", "V"], ["71", "TelPMD6Vp45VAVG", "32.268", "V"], ["72", "TelPMD6Vp45VMax", "32.279", "V"], ["73", "TelPMD6Vn45VMin", "-32.858", "V"], ["74", "TelPMD6Vn45VAVG", "-32.809", "V"], ["75", "TelPMD6Vn45VMax", "-32.702", "V"], ["76", "TelPMD6Vp8VMin", "8.004", "V"], ["77", "TelPMD6Vp8VAVG", "8.026", "V"], ["78", "TelPMD6Vp8VMax", "8.039", "V"], ["79", "TelPMD6Vp5VMin", "5.151", "V"], ["80", "TelPMD6Vp5VAVG", "5.161", "V"], ["81", "TelPMD6Vp5VMax", "5.170", "V"], ["82", "TelPMD6Vp20VMin", "17.595", "V"], ["83", "TelPMD6Vp20VAVG", "17.648", "V"], ["84", "TelPMD6Vp20VMax", "17.684", "V"], ["85", "TelPMD6Vn8VMin", "-8.294", "V"], ["86", "TelPMD6Vn8VAVG", "-8.277", "V"], ["87", "TelPMD6Vn8VMax", "-8.259", "V"], ["88", "TelPMD6Vn20VMin", "-17.705", "V"], ["89", "TelPMD6Vn20VAVG", "-17.641", "V"], ["90", "TelPMD6Vn20VMax", "-17.595", "V"], ["91", "TelPMD6VRefIntMin", "1.198", "V"], ["92", "TelPMD6VRefIntAVG", "1.200", "V"], ["93", "TelPMD6VRefIntMax", "1.202", "V"], ["94", "TelPMD6TempSensor", "40.1", "°C"], ["95", "TelPMPassPacketCount", "25814", ""], ["96", "TelPMErrorPacketCount", "242", ""]]
  in  "ReadTelem":bool
  in  "Telemetry":string(combo) caption="Table"
  in  "Номер параметра 2":i32
  out "float number":sgl
  out "NParam":i32
  in  "ReadOneInt":bool
  out "TableInt":string[][](table)=[["1", "Режим сканирования", "0", ""], ["2", "Состояние ЭБ НЧ", "0", ""], ["3", "Номер датчика для возбуждения", "0", ""], ["4", "Количество усреднений принятых эхосигналов", "1", ""], ["5", "ФНЧ приемников", "0", "кГц"], ["6", "ФВЧ приемников", "0", "кГц"], ["7", "Режим работы узла ВРЧ", "0", ""], ["8", "Тип и версия ПЛИС", "1510473728", ""], ["9", "Дата сборки ПО ПЛИС", "1705238133", "UNIX Time"], ["10", "Дата сборки ПО МК мониторинга платы АЦП", "1699862462", "UNIX Time"], ["11", "Дата сборки ПО МК мониторинга ИП D2", "1698854462", "UNIX Time"], ["12", "Дата сборки ПО МК мониторинга ИП D6", "1698852938", "UNIX Time"], ["13", "IP адрес электронного блока по умолчанию", "-1191073600", "IPv4"], ["14", "Маска подсети", "16777215", "IPv4"], ["15", "Основной шлюз ", "16885952", "IPv4"], ["16", "Сохранение параметров", "0", ""]]
  out "Номер параметра":i32
  in  "Значение параметра":i32
  in  "ReadAllInt":bool
  in  "WriteOneInt":bool
  in  "Int":string(combo)
  in  "ReadDescFloat":bool
  in  "TableFloat":string[][](table)=[["1", "Частота повторения импульсов возбуждения", " 20,000000", "Гц"], ["2", "Частота сигнала заполнения импульса возбуждения", " 40,000000", "кГц"], ["3", "Количество периодов заполнения импульса возбуждения", " 10,000000", "шт"], ["4", "Амплитуда импульса возбуждения", " 100,000000", "%"], ["5", "Задержка начала импульса возбуждения", " 0,000000", "мкс"], ["6", "Задержка области сканирования", " 0,000000", "мкс"], ["7", "Длительность области сканирования", " 100,800003", "мкс"], ["8", "Частота дискретизации сигнала принимаемого с ПЭП сигнала", " 1041666,687500", "Гц"], ["9", "Начальное значение коэффициента усиления приемников", " 0,000172", "дБ"], ["10", "Скорость изменения чувствительности", " 0,000000", "дБ/мс"]]
  in  "ReadAllFloat":bool
  in  "WriteOneFloat":bool
  in  "ReadOneFloat":bool
  in  "Float":string(combo)
  in  "ParamIn":sgl
  out "NumParam":i32
  in  "ReadDescTable":bool
  in  "TableIndex":u8
  out "Waveform Graph":sgl[](graph)
  out "Table":sgl[][][](array[numeric])=[[[0.0, 1.0], [0.0, 1.0], [0.0, 1.0], [0.0, 1.0], [0.0, 1.0], [0.0, 1.0], [0.0, 1.0], [0.0, 1.0], [0.0, 1.0], [0.0, 1.0], [0.0, 1.0], [0.0, 1.0], [0.0, 1.0], [0.0, 1.0], [0.0, 1.0], [0.0, 1.0]]]
  in  "NTable":i32=1
  in  "ReadTable":bool
  in  "Table 2":string(combo) caption="Table"
  in  "NumRead":i32=1
  out "NumGoodRead":i32
  out "sum":i32
  out "output cluster":T11
  in  "PrepTable":bool
  in  "ProgTable":bool
  in  "ReleaseTable":bool
  in  "Param 2":cluster{"Номер табличного параметра":i32}
  in  "Param":cluster{"Номер табличного параметра":i32}
  out "Номер табличного параметра":i32
  out "Cluster":T12
  in  "PrepTable 2":T13 {"Номер колонки" min=0 step=4}
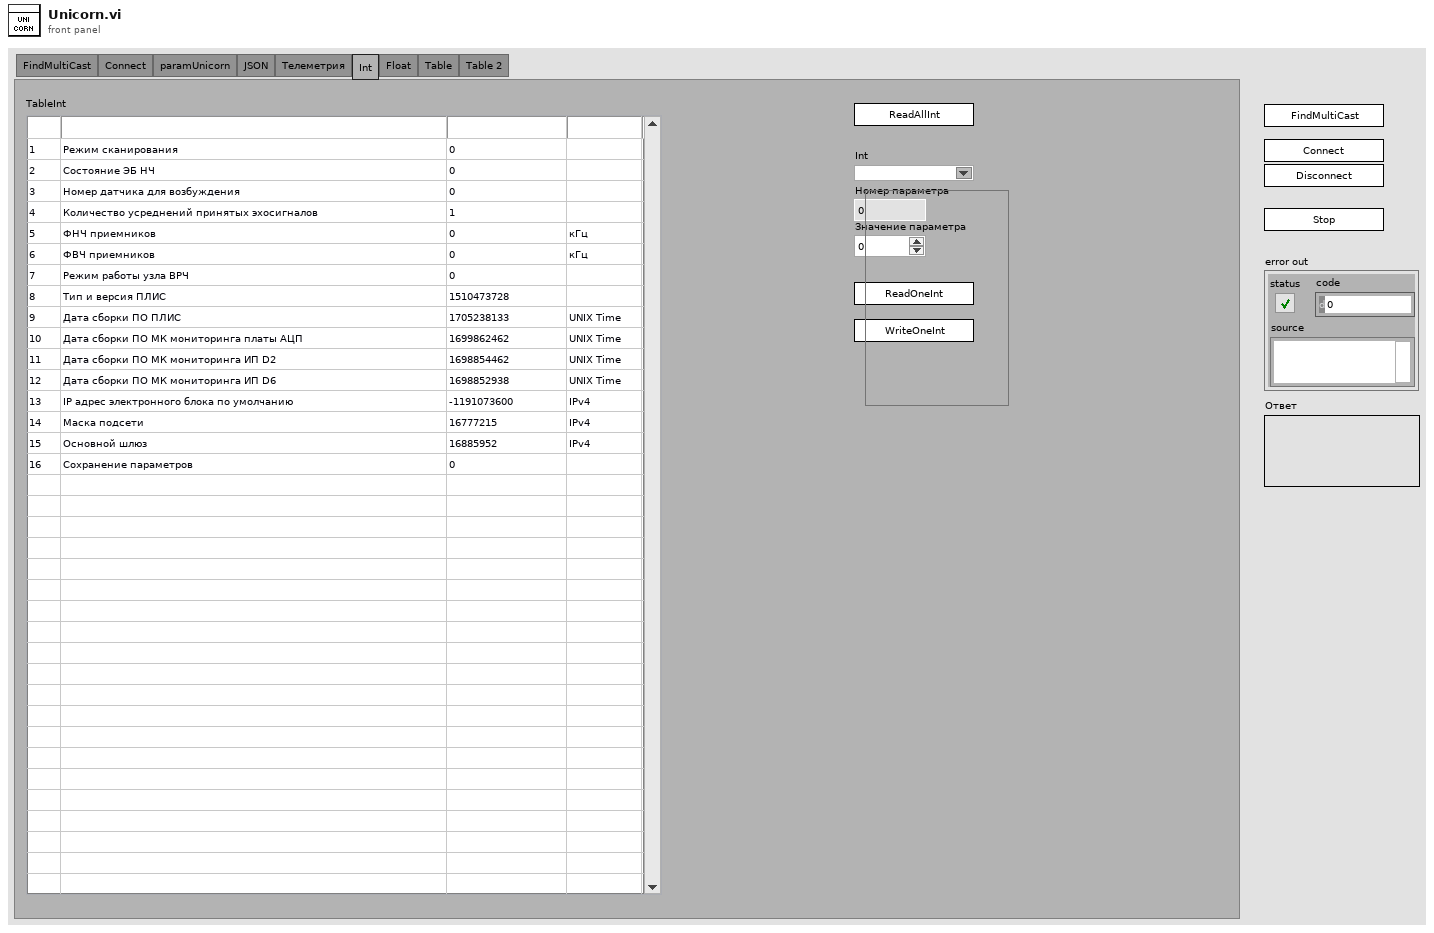
[diagram p1: front panel]
types:
  T1 = enum32{"FindMultiCast", "Connect", "paramUnicorn", "JSON", "Телеметрия", "Int", "Float", "Table", "Table 2"}
  T2 = typedef "LV_Unicorn.lvlib/AnswerUDP.ctl" = cluster{"IP":string, "Port":u16, "DataVersion":u16, "ModbusAddress":i32, "type_version":string, "Description":string, "Serial":string, "ServerPort":u16}
  T3 = typedef "LV_Unicorn.lvlib/unicorn_array.ctl" = cluster{"ArrayInt":i32[], "ArrayFloat":sgl[], "Telemetry":sgl[]}
  T4 = typedef "LV_Unicorn.lvlib/unicorn_Param.ctl" = cluster{"conParam":T5, "Param":T6}
  T5 = typedef "LV_Unicorn.lvlib/unicorn_conn.ctl" = cluster{"ReadIntParam":bool, "ReadDescrParam":bool, "ReadFloatParam":bool, "debug":bool, "ReadJSON":bool, "IP_address":string, "N_attempts":i32, "type_con":enum16{"Serial", "TCP"}, "MB_address":i32, "VISA":refnum<visa-resource-name>, "connection ID":refnum<k5>, "nameDevices":string, "timeout":i32, "port":u16, "type_version":string, "baud_rate":u32, "VersionControl":bool, "TCP_conn":bool, "WindowSize":i32}
  T6 = typedef "LV_Unicorn.lvlib/unicorn_JSON.ctl" = cluster{"NumParam":cluster{"NTelem":i32, "NInt":i32, "NFloat":i32, "NTable":i32}, "ParamInt":T7, "Telemetry":T8, "Table":T9, "ParamFloat":T10}
  T7 = typedef "LV_Unicorn.lvlib/unicorn_ParamInt.ctl" = cluster{"ID":string, "Num":i32, "Name":string, "Type":string, "Enum":string, "Desc":string, "Unit":string, "Access":string, "FormatStr":string, "Min":i32, "Max":i32}[]
  T8 = typedef "LV_Unicorn.lvlib/unicorn_Telemetry.ctl" = cluster{"ID":string, "Num":i32, "Name":string, "Desc":string, "Unit":string, "FormatStr":string, "Min":i32, "Max":i32}[]
  T9 = typedef "LV_Unicorn.lvlib/unicorn_Table.ctl" = cluster{"Num":i32, "Access":string, "ColumnCount":i32, "NeedParamPrepare":bool, "Columns":cluster{"Column":i32, "Desc":string, "Name":string}[], "DataType":string, "FormatStr":string, "ID":string, "Name":string, "RowCount":i32, "Rows":cluster{"Desc":string, "ID":string, "Max":i32, "Min":i32, "Name":string, "Row":i32, "Unit":string}[], "Type":string}[]
  T10 = typedef "LV_Unicorn.lvlib/unicorn_ParamFloat.ctl" = cluster{"ID":string, "Num":i32, "Name":string, "Type":string, "Enum":string, "Desc":string, "Unit":string, "Access":string, "FormatStr":string, "Min":sgl, "Max":sgl}[]
  T11 = cluster{"Int":refnum<vi>, "Float":refnum<vi>, "Table":refnum<vi>, "Telemetry":refnum<vi>}
  T12 = cluster{"Номер табличного параметра":i32, "Количество пройденных шагов (прогресс)":i32, "Общее количество шагов для получения результата":i32, "Количество строк в подготовленном табличном параметре":i32, "Количество столбцов в подготовленном табличном параметре":i32}
  T13 = cluster{"Режим":i32, "Номер табличного параметра":i32, "Номер колонки":i32}
  T14 = cluster{"NumTable":i32, "Progress":i32, "Общее количество шагов для получения результата":i32, "Количество строк в подготовленном табличном параметре":i32, "Количество столбцов в подготовленном табличном параметре":i32}
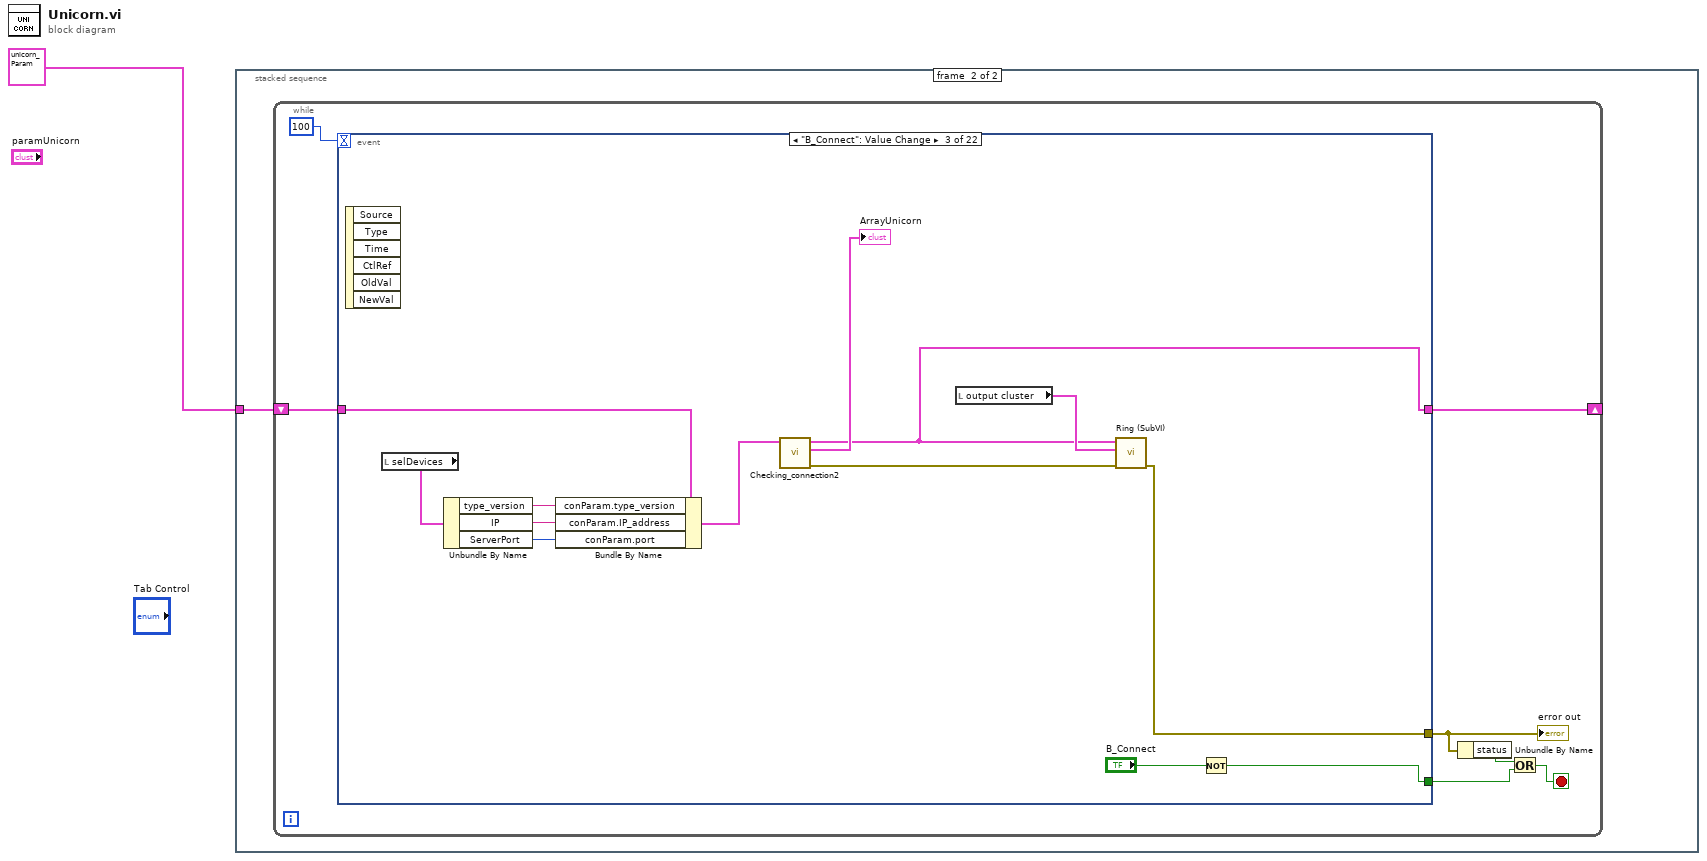
[diagram p0: block diagram]
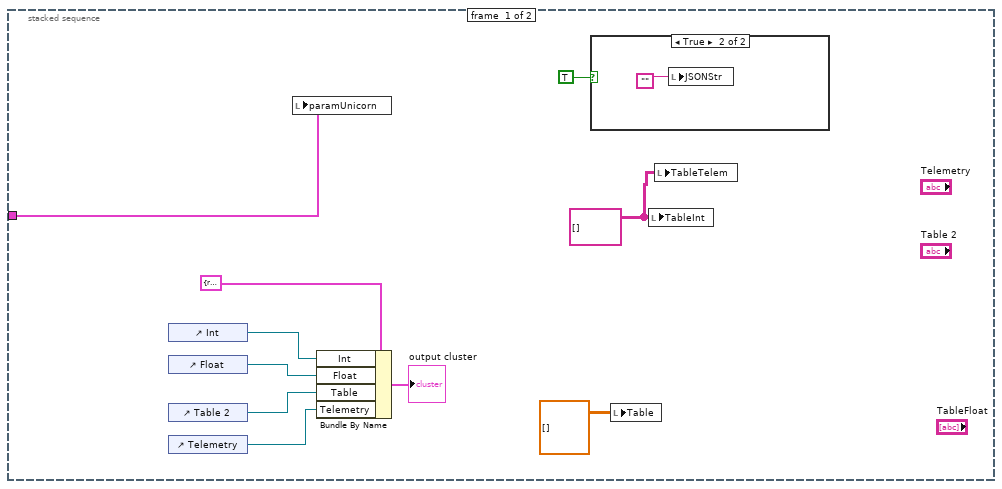
[diagram p2: hidden frame]
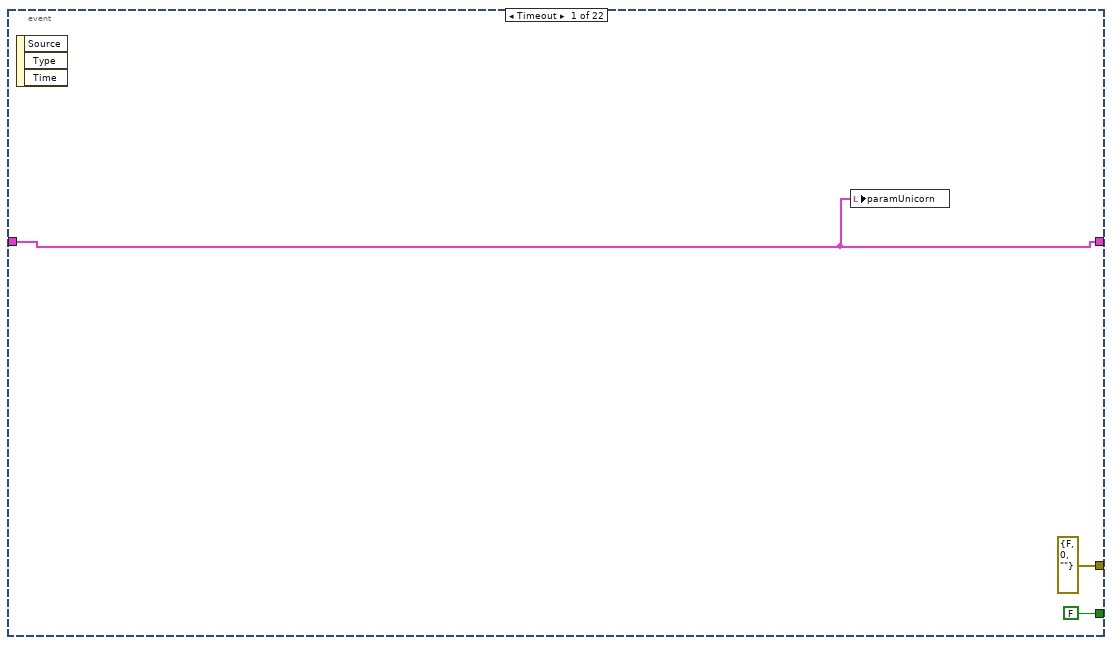
[diagram p4: hidden frame]
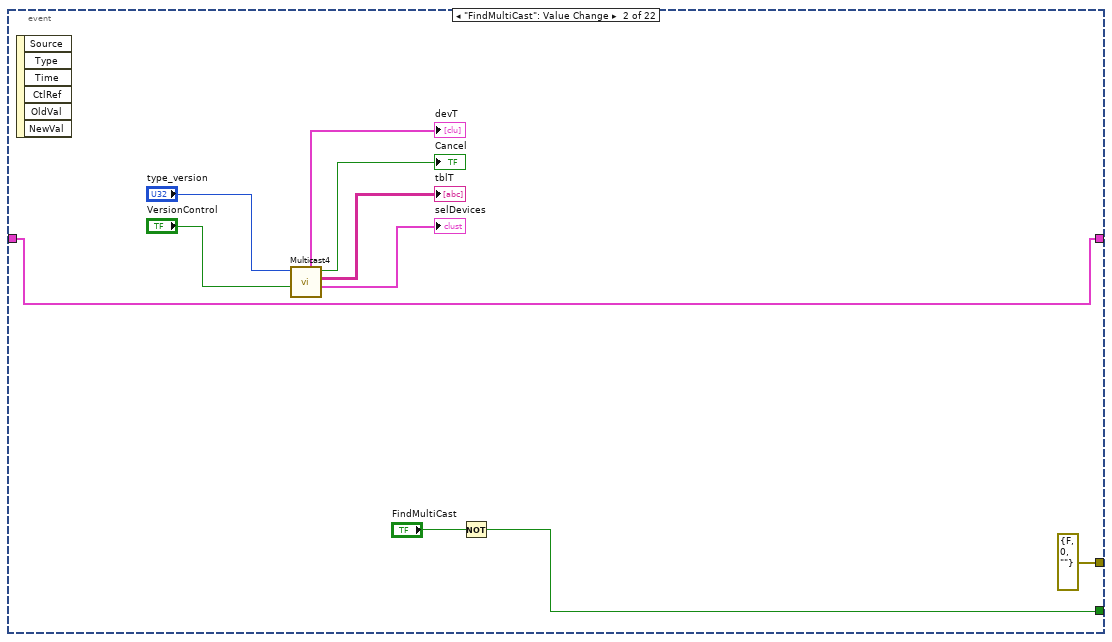
[diagram p5: hidden frame]
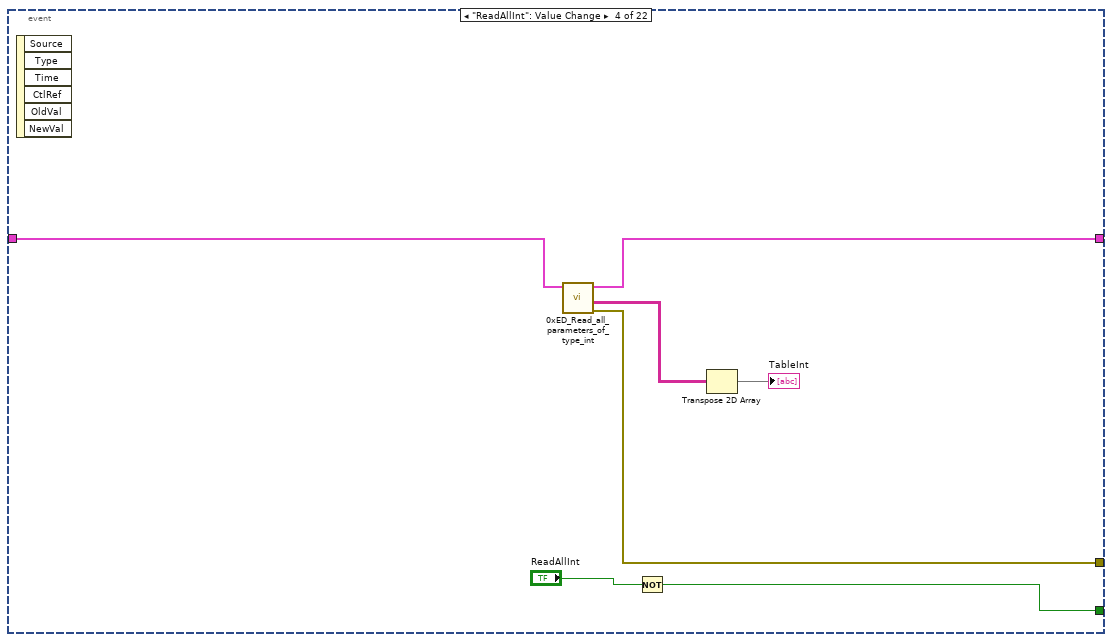
[diagram p6: hidden frame]
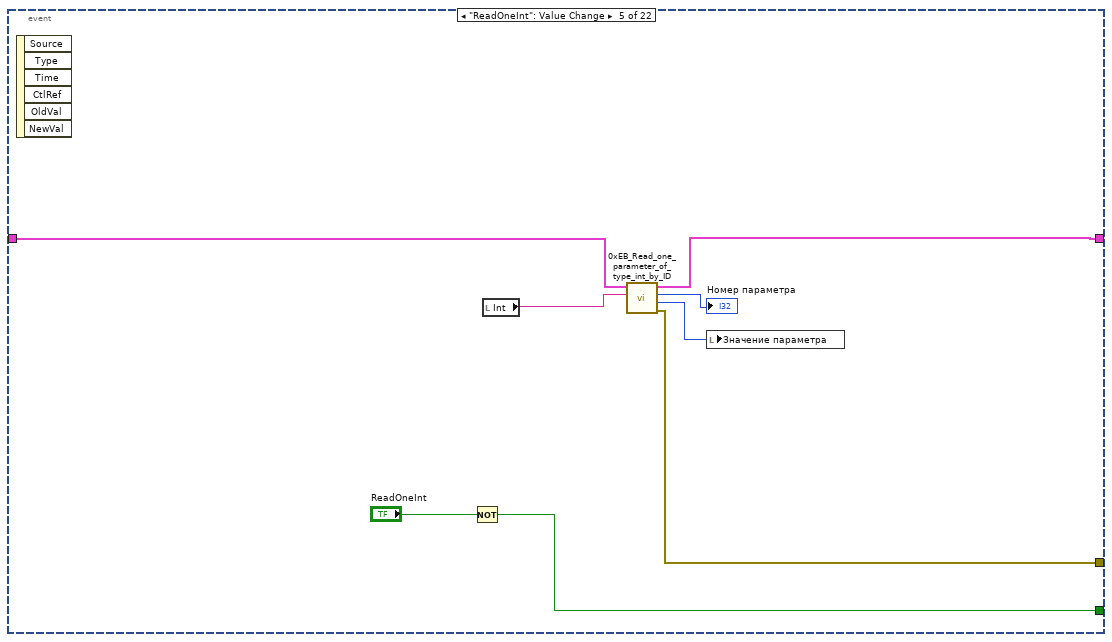
[diagram p7: hidden frame]
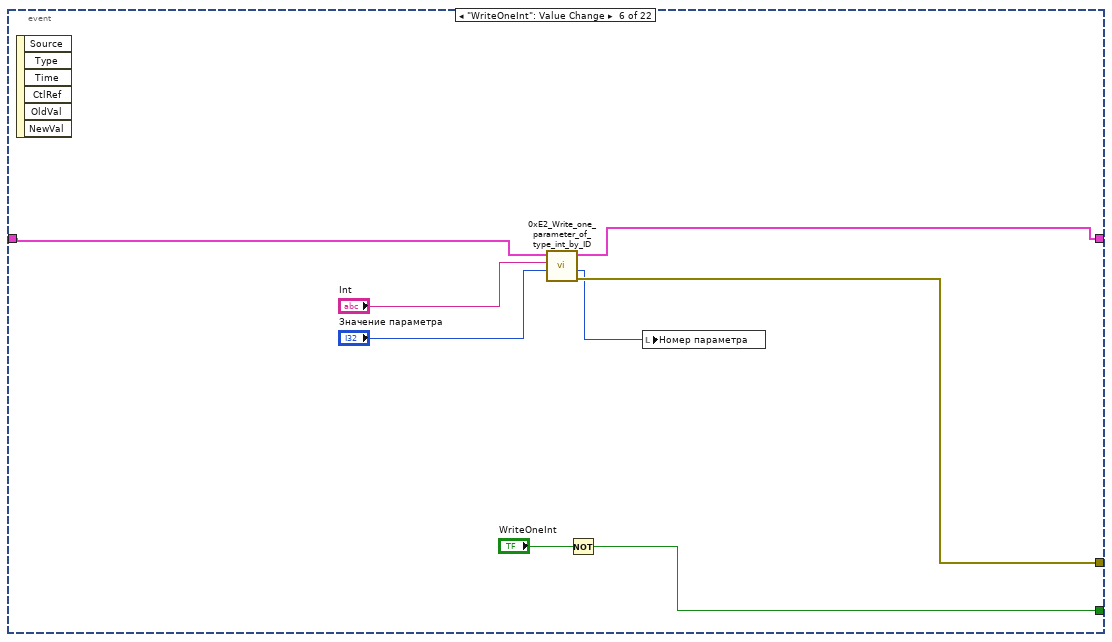
[diagram p8: hidden frame]
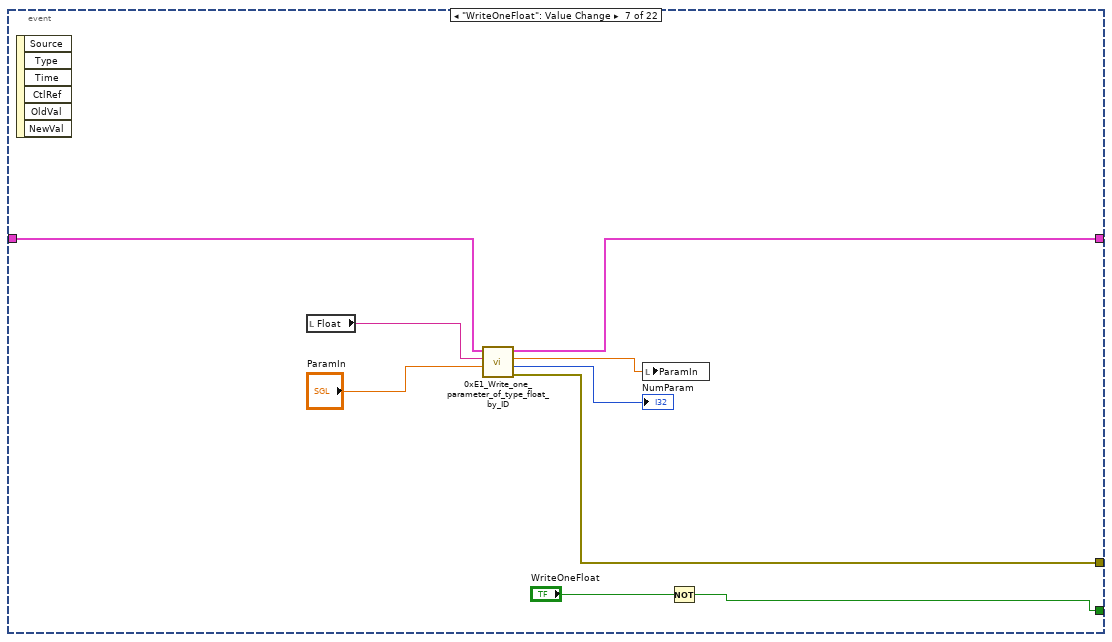
[diagram p9: hidden frame]
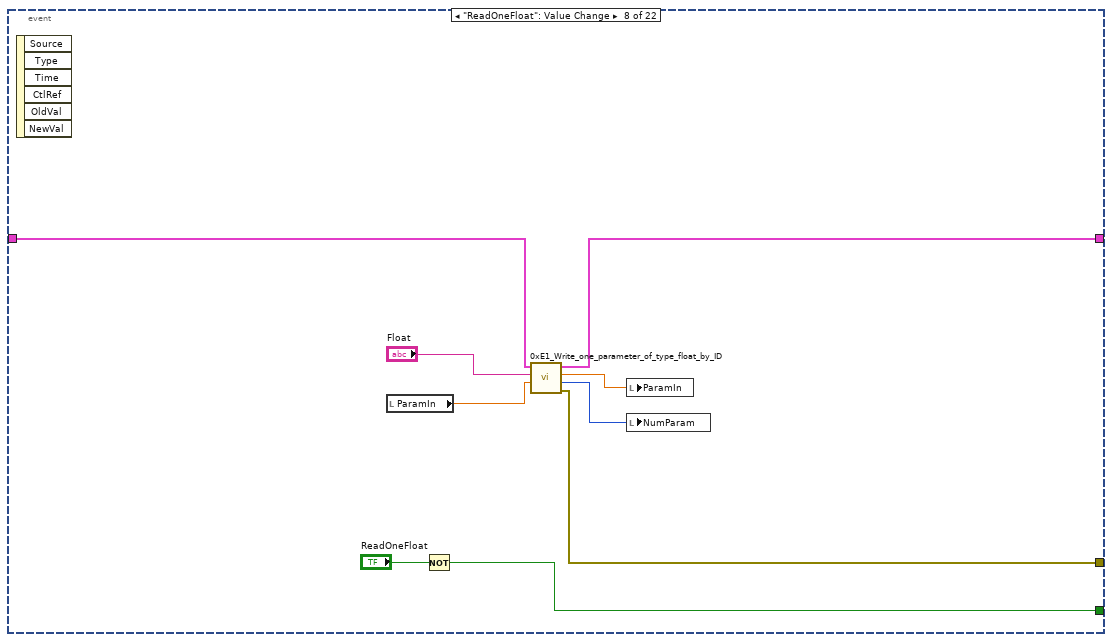
[diagram p10: hidden frame]
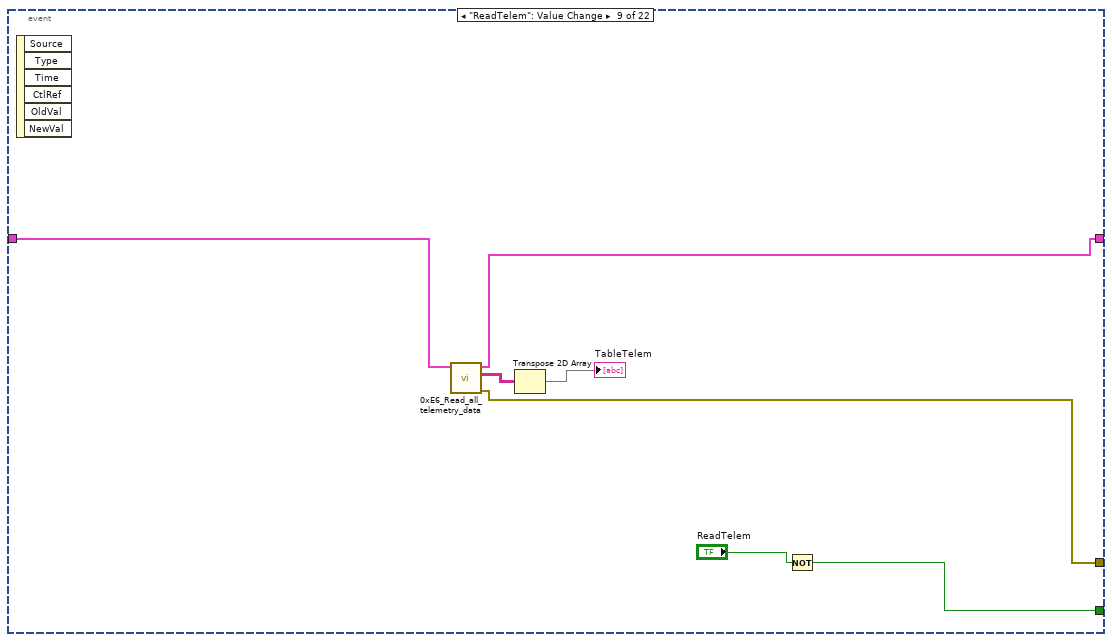
[diagram p11: hidden frame]
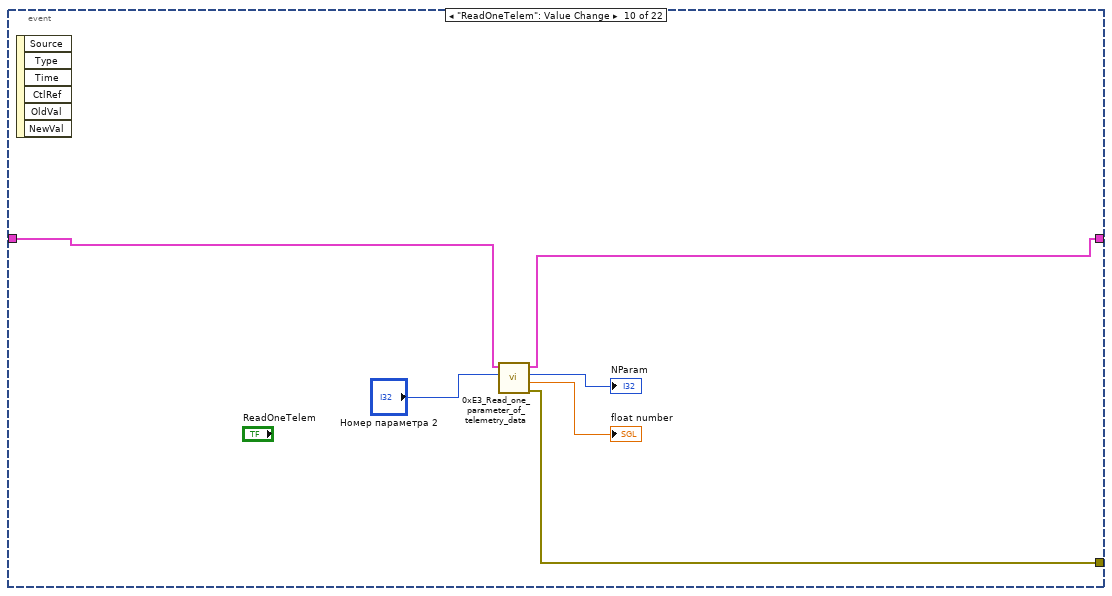
[diagram p12: hidden frame]
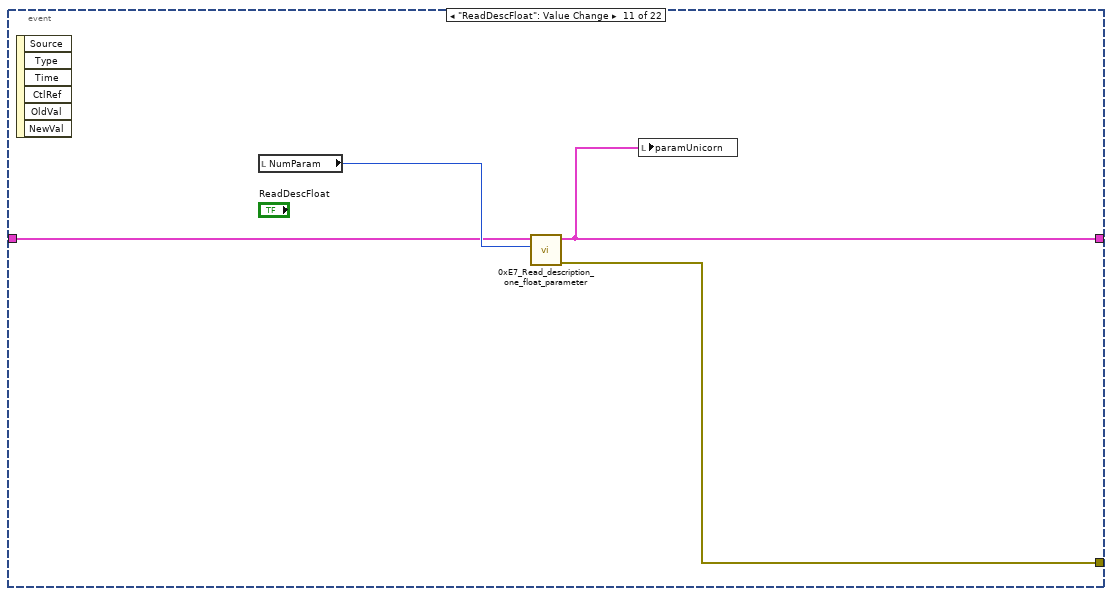
[diagram p13: hidden frame]
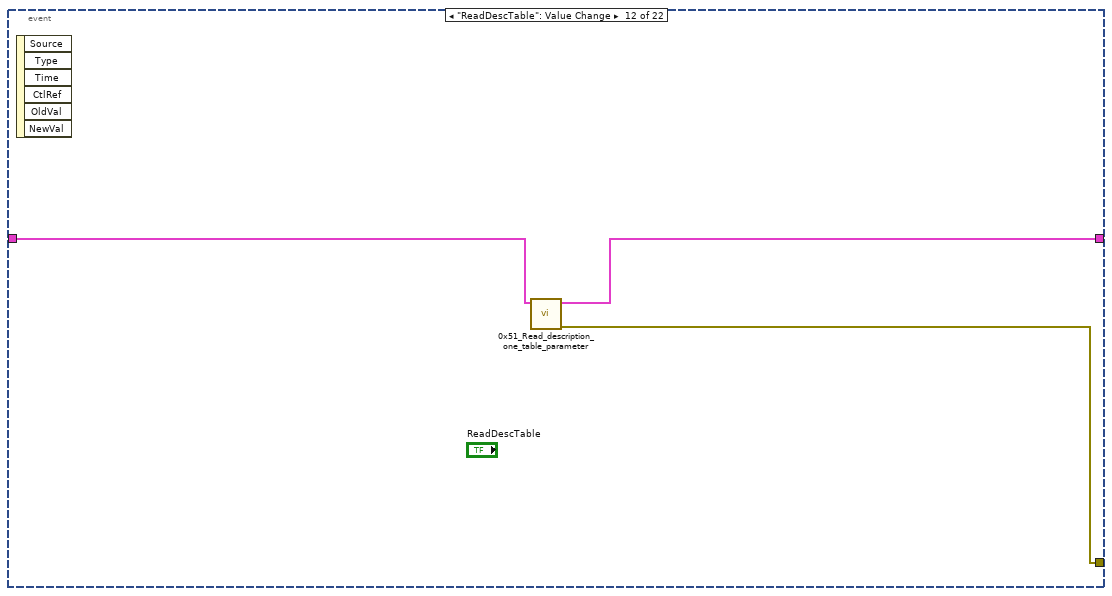
[diagram p14: hidden frame]
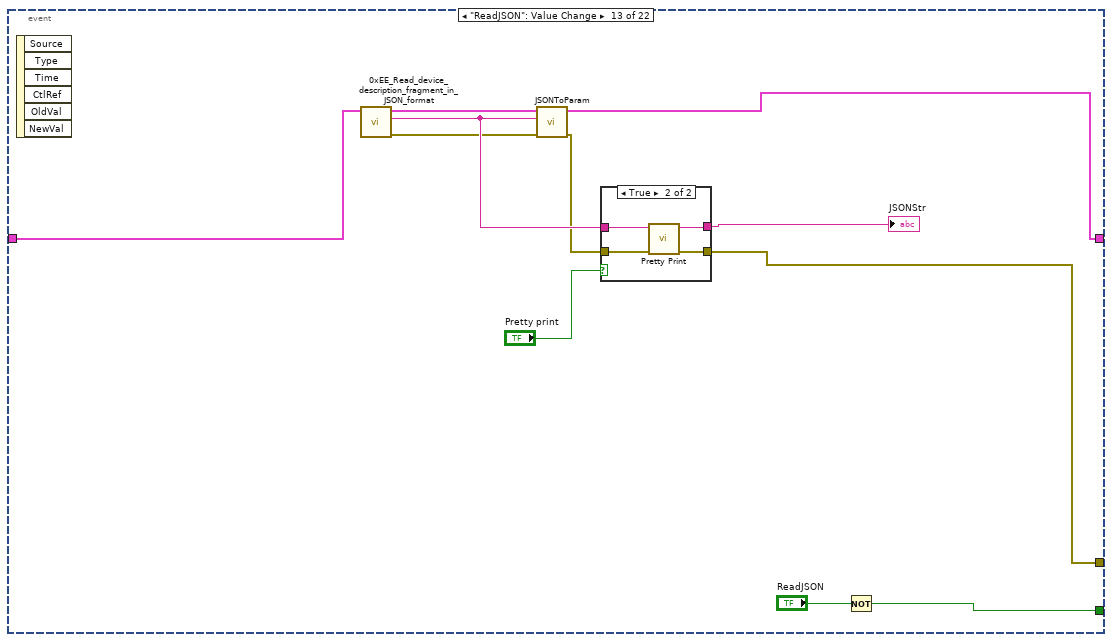
[diagram p15: hidden frame]
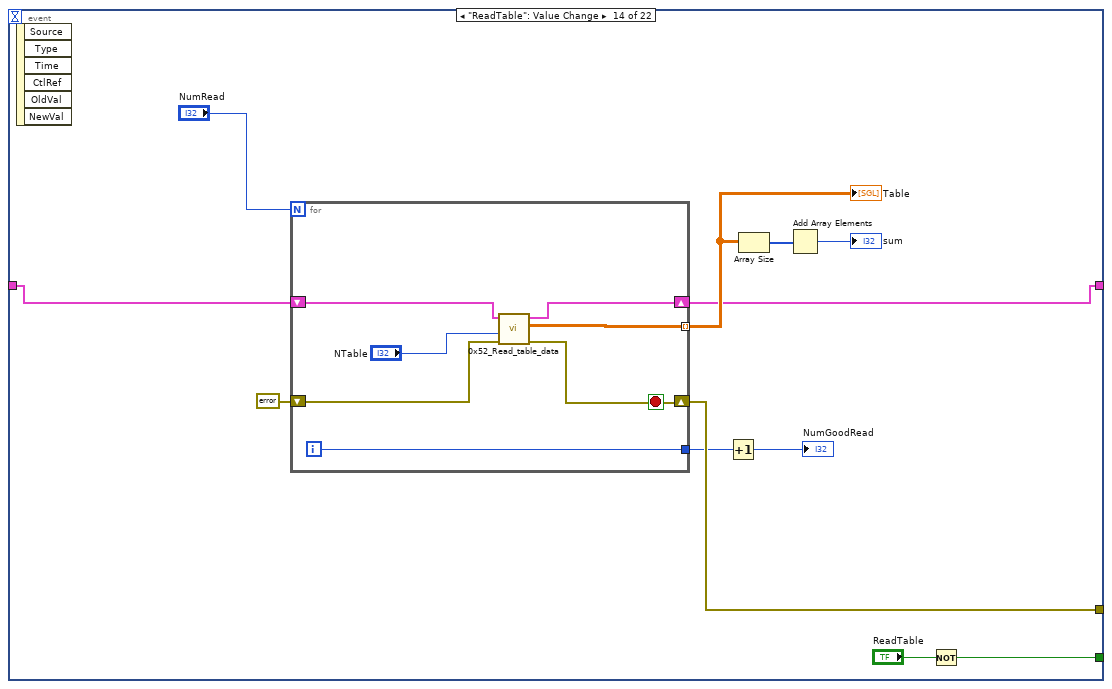
[diagram p17: hidden frame]
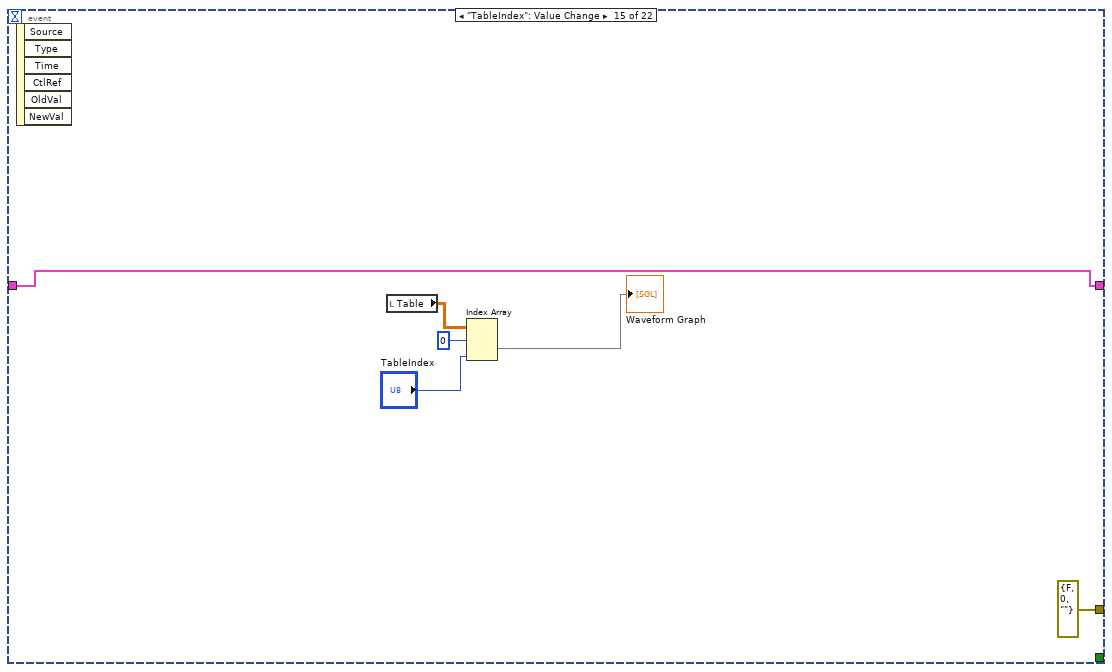
[diagram p18: hidden frame]
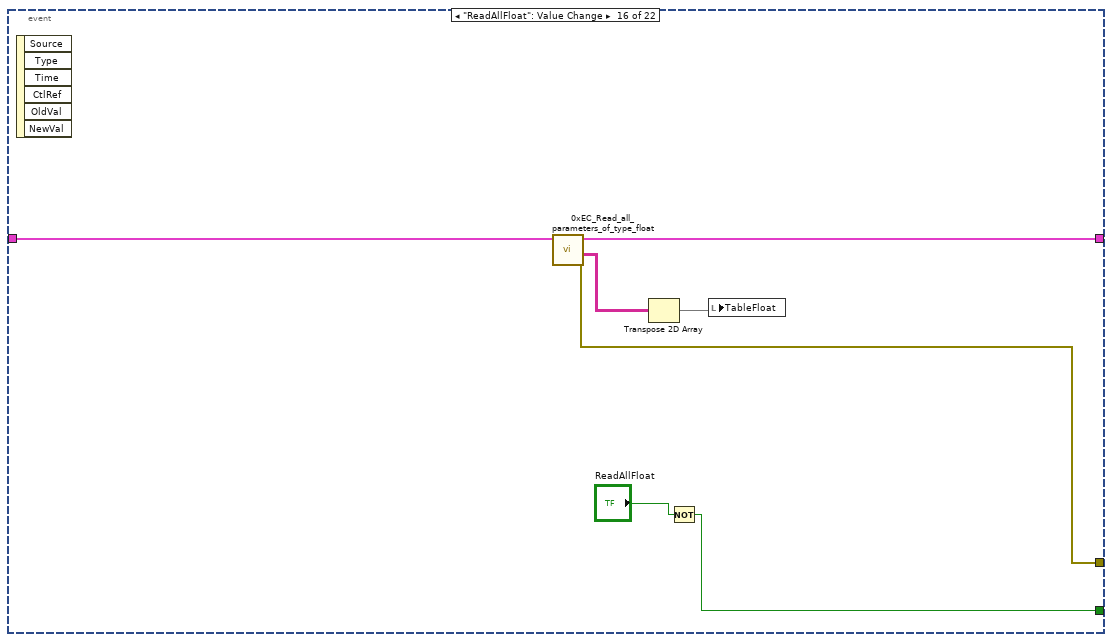
[diagram p19: hidden frame]
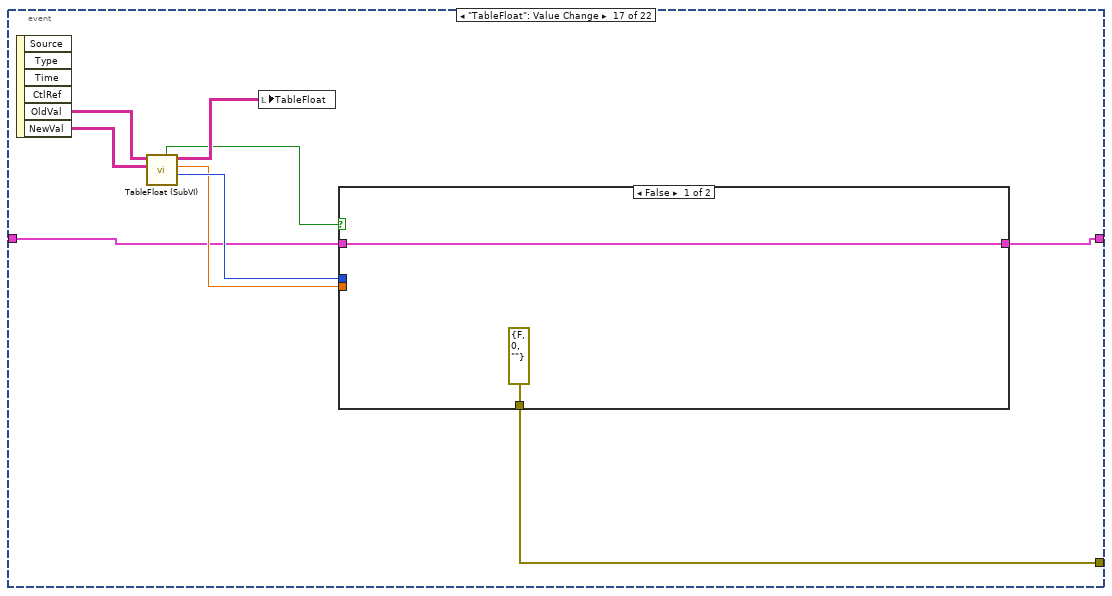
[diagram p20: hidden frame]
diagram:
  n1 = stacked-sequence {
    tunnel: T4 {"conParam"={"ReadIntParam"=TRUE, "ReadDescrParam"=FALSE, "ReadFloatParam"=TRUE, "debug"=FALSE, "ReadJSON"=TRUE, "IP_address"="192.168.1.216", "N_attempts"=3, "type_con"=enum."TCP", "MB_address"=1, "VISA"="COM1", "connection ID"=refnum, "nameDevices"="", "timeout"=1000, "port"=2000, "type_version"="0F0C0001", "baud_rate"=115200, "VersionControl"=TRUE, "TCP_conn"=FALSE, "WindowSize"=700}, "Param"={"NumParam"={"NTelem"=201, "NInt"=16, "NFloat"=10, "NTable"=2}, "ParamInt"=[{"ID"="Режим работы", "Num"=0, "Name"="", "Type"="", "Enum"="", "Desc"="", "Unit"="", "Access"="", "FormatStr"="", "Min"=0, "Max"=0}, {"ID"="", "Num"=0, "Name"="", "Type"="", "Enum"="", "Desc"="", "Unit"="", "Access"="", "FormatStr"="", "Min"=0, "Max"=0}, {"ID"="", "Num"=0, "Name"="", "Type"="", "Enum"="", "Desc"="", "Unit"="", "Access"="", "FormatStr"="", "Min"=0, "Max"=0}, {"ID"="", "Num"=0, "Name"="", "Type"="", "Enum"="", "Desc"="", "Unit"="", "Access"="", "FormatStr"="", "Min"=0, "Max"=0}, {"ID"="", "Num"=0, "Name"="", "Type"="", "Enum"="", "Desc"="", "Unit"="", "Access"="", "FormatStr"="", "Min"=0, "Max"=0}, {"ID"="", "Num"=0, "Name"="", "Type"="", "Enum"="", "Desc"="", "Unit"="", "Access"="", "FormatStr"="", "Min"=0, "Max"=0}, {"ID"="ModeWork", "Num"=0, "Name"="", "Type"="", "Enum"="", "Desc"="", "Unit"="", "Access"="", "FormatStr"="", "Min"=0, "Max"=0}], "Telemetry"=[], "Table"=[], "ParamFloat"=[]}} ("paramUnicorn") -> [w3 w13]
    frame #0 {
      w11 = string[][] [] ("Таблица int")
      n2 = control-ref of="Int"() -> (w8:refnum<vi>)
      n3 = control-ref of="Float"() -> (w7:refnum<vi>)
      n4 = control-ref of="Table 2"() -> (w6:refnum<vi>)
      n5 = control-ref of="Telemetry"() -> (w5:refnum<vi>)
      n6 = local write "paramUnicorn"(w3) -> ()
      n7 = Bundle By Name(cluster=T11 {"Int"=refnum, "Float"=refnum, "Table"=refnum, "Telemetry"=refnum} ("Ref"), "Int"=w8, "Float"=w7, "Table"=w6, "Telemetry"=w5) -> (→"output cluster":T11)
      n8 = case shown="True" TRUE {
        frame False {
        }
        frame True {
          n9 = local write "JSONStr"("") -> ()
        }
      }
      n10 = local write "Table"(sgl[][][] [] ("Array 3")) -> ()
      n11 = local write "TableInt"(w11) -> ()
      n12 = local write "TableTelem"(w11) -> ()
    }
    frame #1 {
      n13 = while {
        shift-right: [w14] -> _
        shift-left: w13 -> [w15]
        stop <- w16 stop-if-true
        n14 = event shown="[2] \"B_Connect\": Value Change" {
          selector: _ -> [_ _ _ _ _ _ _ _ _ _ _ _ _ _ _ _ _ _ _ _ _ _]
          dyn-events: _ -> [_ _ _ _ _ _ _ _ _ _ _ _ _ _ _ _ _ _ _ _ _ _]
          timeout: 100 -> [_ _ _ _ _ _ _ _ _ _ _ _ _ _ _ _ _ _ _ _ _ _]
          tunnel: [FALSE ("B_Stop") w32 w41 w52 w56 w68 w73 w81 w93 _ _ _ w117 w135 _ w153 _ w176 w187 w199 "B_Stop" w215] -> w17
          tunnel: [errorcluster {"status"=FALSE, "code"=0, "source"=""} ("error out") errorcluster {"status"=FALSE, "code"=0, "source"=""} ("error out") w36 w51 w58 w67 w72 w83 w92 w95 w102 w105 w116 w134 errorcluster {"status"=FALSE, "code"=0, "source"=""} ("error out") w156 w157 w178 w189 w201 errorcluster {"status"=FALSE, "code"=0, "source"=""} ("error out") w214] -> w19
          tunnel: [w21 w24 w34 w48 w55 w62 w70 w79 w88 w96 w103 w106 w108 w126 w145 w150 w158 w175 w186 w198 w209 w212] -> w14
          tunnel: w15 -> [w21 w24 w35 w47 w54 w63 w71 w80 w89 w97 w101 w107 w109 w127 w145 w151 w159 w175 w186 w198 w209 w213]
          event Timeout {
            n15 = event-data() -> ()  [unwired: 1 in, 3 out]
            n16 = local write "paramUnicorn"(w21) -> ()
          }
          event "FindMultiCast": Value Change {
            n17 = event-data() -> ()  [unwired: 1 in, 6 out]
            n18 = call "Multicast4.vi"("VersionControl"="VersionControl", "type_version"="type_version") -> ("selDevice"=→"selDevices":T2, "tblT"=→"tblT":string[][], "Cancel"=→"Cancel":bool, "foundDevices"=→"devT":T2[])  [unwired: 4 in, 2 out]
            n19 = Not(x="FindMultiCast") -> (.not. x?=w32:bool)
          }
          event "B_Connect": Value Change {
            n20 = event-data() -> ()  [unwired: 1 in, 6 out]
            n21 = local read "selDevices"() -> (w46:T2)
            n22 = Unbundle By Name(w46) -> ("type_version"=w40:string, "IP"=w45:string, "ServerPort"=w39:u16)
            n23 = Bundle By Name(cluster=w35, "conParam.type_version"=w40, "conParam.IP_address"=w45, "conParam.port"=w39) -> (w44:T4)
            n24 = call "Checking_connection2.vi"("paramUnicornIn"=w44) -> ("error out"=w37:errorcluster, "ArrayData"=→"ArrayUnicorn":T3, "paramUnicorn"=w34:T4)  [unwired: 7 in, 1 out]
            n25 = local read "output cluster"() -> (w38:T11)
            n26 = call "Ring (SubVI).vi"("error in"=w37, "Ref"=w38, "paramUnicorn"=w34) -> ("error out"=w36:errorcluster)  [unwired: 8 in]
            n27 = Not(x="B_Connect") -> (.not. x?=w41:bool)
          }
          event "ReadAllInt": Value Change {
            n28 = event-data() -> ()  [unwired: 1 in, 6 out]
            n29 = call "0xED_Read_all_parameters_of_type_int.vi"("paramUnicorn"=w47) -> ("error out"=w51:errorcluster, "ArrayIntStr"=w50:string[][], "paramUnicorn 2"=w48:T4)  [unwired: 7 in, 1 out]
            n30 = Not(x="ReadAllInt") -> (.not. x?=w52:bool)
            n31 = Transpose 2D Array(2D array=w50) -> (transposed array=→"TableInt":string[][])
          }
          event "ReadOneInt": Value Change {
            n32 = event-data() -> ()  [unwired: 1 in, 6 out]
            n33 = Not(x="ReadOneInt") -> (.not. x?=w56:bool)
            n34 = local read "Int"() -> (w61:string)
            n35 = call "0xEB_Read_one_parameter_of_type_int_by_ID.vi"("ID_IntParam"=w61, "paramUnicorn"=w54) -> ("error out"=w58:errorcluster, "Значение параметра"=w60:i32, "Номер параметра"=→"Номер параметра":i32, "ParamOut"=w55:T4)  [unwired: 6 in]
            n36 = local write "Значение параметра"(w60) -> ()
          }
          event "WriteOneInt": Value Change {
            n37 = event-data() -> ()  [unwired: 1 in, 6 out]
            n38 = call "0xE2_Write_one_parameter_of_type_int_by_ID.vi"("ParamIn"="Значение параметра", "ID_IntParam"="Int", "paramUnicorn"=w63) -> ("error out"=w67:errorcluster, "NumParam"=w64:i32, "paramUnicornOut"=w62:T4)  [unwired: 6 in]
            n39 = Not(x="WriteOneInt") -> (.not. x?=w68:bool)
            n40 = local write "Номер параметра"(w64) -> ()
          }
          event "WriteOneFloat": Value Change {
            n41 = event-data() -> ()  [unwired: 1 in, 6 out]
            n42 = local read "Float"() -> (w78:string)
            n43 = call "0xE1_Write_one_parameter_of_type_float_by_ID.vi"("ParamIn"="ParamIn", "ID_floatParam"=w78, "paramUnicorn"=w71) -> ("error out"=w72:errorcluster, "NumParam"=→"NumParam":i32, "ParamOut"=w75:sgl, "paramUnicornOut"=w70:T4)  [unwired: 5 in]
            n44 = local write "ParamIn"(w75) -> ()
            n45 = Not(x="WriteOneFloat") -> (.not. x?=w73:bool)
          }
          event "ReadOneFloat": Value Change {
            n46 = event-data() -> ()  [unwired: 1 in, 6 out]
            n47 = local read "ParamIn"() -> (w84:sgl)
            n48 = Not(x="ReadOneFloat") -> (.not. x?=w81:bool)
            n49 = call "0xE1_Write_one_parameter_of_type_float_by_ID.vi"("ParamIn"=w84, "ID_floatParam"="Float", "paramUnicorn"=w80) -> ("error out"=w83:errorcluster, "NumParam"=w85:i32, "ParamOut"=w86:sgl, "paramUnicornOut"=w79:T4)  [unwired: 5 in]
            n50 = local write "ParamIn"(w86) -> ()
            n51 = local write "NumParam"(w85) -> ()
          }
          event "ReadTelem": Value Change {
            n52 = event-data() -> ()  [unwired: 1 in, 6 out]
            n53 = call "0xE6_Read_all_telemetry_data.vi"("paramUnicorn"=w89) -> ("error out"=w92:errorcluster, "TblTelemetry"=w90:string[][], "paramUnicorn 2"=w88:T4)  [unwired: 6 in, 1 out]
            n54 = Transpose 2D Array(2D array=w90) -> (transposed array=→"TableTelem":string[][])
            n55 = Not(x="ReadTelem") -> (.not. x?=w93:bool)
          }
          event "ReadOneTelem": Value Change {
            n56 = event-data() -> ()  [unwired: 1 in, 6 out]
            n57 = call "0xE3_Read_one_parameter_of_telemetry_data.vi"("Номер параметра"="Номер параметра 2", "ParamIn"=w97) -> ("error out"=w95:errorcluster, "float number"=→"float number":sgl, "NParam"=→"NParam":i32, "ParamOut"=w96:T4)  [unwired: 6 in]
          }
          event "ReadDescFloat": Value Change {
            n58 = event-data() -> ()  [unwired: 1 in, 6 out]
            n59 = local read "NumParam"() -> (w104:i32)
            n60 = call "0xE7_Read_description_one_float_parameter.vi"("NumberFloatParam"=w104, "paramUnicornIn in"=w101) -> ("error out"=w102:errorcluster, "paramUnicornIn out 2"=w103:T4)  [unwired: 6 in, 2 out]
            n61 = local write "paramUnicorn"(w103) -> ()
          }
          event "ReadDescTable": Value Change {
            n62 = event-data() -> ()  [unwired: 1 in, 6 out]
            n63 = call "0x51_Read_description_one_table_parameter.vi"("paramUnicornIn in"=w107) -> ("error out"=w105:errorcluster, "paramUnicornIn out 2"=w106:T4)  [unwired: 9 in]
          }
          event "ReadJSON": Value Change {
            n64 = event-data() -> ()  [unwired: 1 in, 6 out]
            n65 = call "0xEE_Read_device_description_fragment_in_JSON_format.vi"("paramUnicorn 2"=w109) -> ("error out"=w114:errorcluster, "JSONStr"=w115:string, "paramUnicorn"=w112:T4)  [unwired: 8 in]
            n66 = call "JSONToParam.vi"("error in"=w114, "JSON"=w115, "paramUnicornIn"=w112) -> ("error out"=w110:errorcluster, "paramUnicornOut"=w108:T4)  [unwired: 7 in]
            n67 = case shown="True" "Pretty print" {
              tunnel: w115 -> [w120 w124]
              tunnel: [w120 w123] -> w113
              tunnel: w110 -> [w119 w122]
              tunnel: [w119 w121] -> w116
              frame False {
              }
              frame True {
                n68 = call <vilib>:"Pretty Print.vi"("error in (no error)"=w122, "JSON"=w124) -> ("error out"=w121:errorcluster, "<JSON>"=w123:string)  [unwired: 7 in, 1 out]
              }
            }
            "JSONStr" <- w113
            n69 = Not(x="ReadJSON") -> (.not. x?=w117:bool)
          }
          event "ReadTable": Value Change {
            n70 = event-data() -> ()  [unwired: 1 in, 6 out]
            n71 = for {
              N: "NumRead" -> [_]
              tunnel: [w141] -> w130
              tunnel: [w140] -> w128 mode=indexing
              shift-right: [w138] -> w126
              shift-left: w127 -> [w139]
              shift-right: [w142] -> w134
              shift-left: errorcluster {"status"=FALSE, "code"=0, "source"=""} ("error out") -> [w137]
              i -> [w141]
              stop <- w142 stop-if-true
              n72 = call "0x52_Read_table_data.vi"("error in"=w137, "NTable"="NTable", "paramUnicornIn"=w139) -> ("error out"=w142:errorcluster, "Array"=w140:sgl[][], "paramUnicornOut"=w138:T4)  [unwired: 6 in]
            }
            "Table" <- w128
            n73 = Increment(x=w130) -> (x+1=→"NumGoodRead":i32)
            n74 = Array Size(array=w128) -> (size(s)=w132:i32[])
            n75 = Add Array Elements(numeric array=w132) -> (sum=→"sum":i32)
            n76 = Not(x="ReadTable") -> (.not. x?=w135:bool)
          }
          event "TableIndex": Value Change {
            n77 = event-data() -> ()  [unwired: 1 in, 6 out]
            n78 = local read "Table"() -> (w149:sgl[][][])
            n79 = Index Array(array=w149, index (dim 0)=0 ("index (page)"), index (dim 2)="TableIndex") -> (element=→"Waveform Graph":sgl[])  [unwired: 1 in]
          }
          event "ReadAllFloat": Value Change {
            n80 = event-data() -> ()  [unwired: 1 in, 6 out]
            n81 = call "0xEC_Read_all_parameters_of_type_float.vi"("paramUnicorn"=w151) -> ("error out"=w156:errorcluster, "ArrayFloatStr"=w155:string[][], "paramUnicorn 2"=w150:T4)  [unwired: 7 in, 1 out]
            n82 = Transpose 2D Array(2D array=w155) -> (transposed array=w152:string[][])
            n83 = Not(x="ReadAllFloat") -> (.not. x?=w153:bool)
            n84 = local write "TableFloat"(w152) -> ()
          }
          event "TableFloat": Value Change {
            n85 = event-data() -> ("OldVal"=w163:string[][], "NewVal"=w165:string[][])  [unwired: 1 in, 4 out]
            n86 = call "TableFloat (SubVI).vi"("NewVal"=w165, "OldVal in"=w163) -> ("NumParam"=w162:i32, "Numeric"=w161:dbl, "OldVal out"=w164:string[][], "ChangeParam"=w160:bool)  [unwired: 6 in]
            n87 = local write "TableFloat"(w164) -> ()
            n88 = case shown="False" w160 {
              tunnel: w162 -> [_ w174]
              tunnel: w161 -> [_ w173]
              tunnel: w159 -> [w167 w170]
              tunnel: [w167 w169] -> w158
              tunnel: [errorcluster {"status"=FALSE, "code"=0, "source"=""} ("error out") w168] -> w157
              frame False {
              }
              frame True {
                n89 = call "0xE1_Write_one_parameter_of_type_float.vi"("Значение параметра"=w173, "Номер параметра"=w174, "ParamIn"=w170) -> ("error out"=w168:errorcluster, "Значение параметра 2"=w172:sgl, "Номер параметра 2"=w171:i32, "ParamOut"=w169:T4)  [unwired: 5 in]
                n90 = local write "NumParam"(w171) -> ()
                n91 = local write "ParamIn"(w172) -> ()
              }
            }
          }
          event "PrepTable": Value Change {
            n92 = event-data() -> ()  [unwired: 1 in, 6 out]
            n93 = disable-structure shown="Disabled" {
              disable-tunnel: [w179 _] -> w178
              frame Disabled {
                n94 = local read item#-1() -> (w180)
                n95 = case shown="False" w180 {
                  tunnel: [w182 _] -> w179
                  frame False {
                    n96 = local read "paramUnicorn"() -> ()  [unwired: 1 out]
                    n97 = call "0x54_Preparing_table_data.vi"("Param"="PrepTable 2") -> ("error out"=w182:errorcluster, "Ответ"=w185:string)  [unwired: 6 in, 3 out]
                    "Ответ" <- w185
                    n98 = local read "paramUnicorn"() -> (w181:T4)
                    n99 = call "Parser_0x54_(SubVI).vi"("String in"=w185) -> ("Номер табличного параметра"=→"Номер табличного параметра":i32)  [unwired: 9 in, 1 out]
                  }
                  frame True {
                  }
                }
              }
              frame Enabled {
              }
            }
            n100 = Not(x="PrepTable") -> (.not. x?=w176:bool)
          }
          event "ProgTable": Value Change {
            n101 = event-data() -> ()  [unwired: 1 in, 6 out]
            n102 = disable-structure shown="Disabled" {
              disable-tunnel: [w191 _] -> w189
              frame Disabled {
                n103 = local read item#-1() -> (w190)
                n104 = case shown="False" w190 {
                  tunnel: [w192 _] -> w191
                  frame False {
                    n105 = local read item#-1() -> (w196)
                    n106 = call "0x55_Progress_preparing_table_data.vi"("Param"="Param", "paramUnicorn 2"=w196) -> ("error out"=w192:errorcluster, "Ответ"=w195:string, "paramUnicorn"=w197:T4)  [unwired: 5 in, 2 out]
                    n107 = local write "Ответ"(w195) -> ()
                    n108 = call "Parser_0x55_(SubVI).vi"("String in"=w195) -> ("Cluster"=→"Cluster":T14)  [unwired: 9 in, 1 out]
                    n109 = local write item#-1(w197) -> ()
                  }
                  frame True {
                  }
                }
              }
              frame Enabled {
              }
            }
            n110 = Not(x="ProgTable") -> (.not. x?=w187:bool)
          }
          event "ReleaseTable": Value Change {
            n111 = event-data() -> ()  [unwired: 1 in, 6 out]
            n112 = disable-structure shown="Disabled" {
              disable-tunnel: [w202 _] -> w201
              frame Disabled {
                n113 = local read item#-1() -> (w203)
                n114 = case shown="False" w203 {
                  tunnel: [w204 _] -> w202
                  frame False {
                    n115 = local read "paramUnicorn"() -> (w207:T4)
                    n116 = call "0x56_Freeing_data_from_a_prepared_table_parameter.vi"("Param"="Param 2") -> ("error out"=w204:errorcluster, "Ответ"=w206:string, "ParamOut"=w208:T5)  [unwired: 7 in, 1 out]
                    n117 = local write "paramUnicorn"(w208) -> ()
                    n118 = local write "Ответ"(w206) -> ()
                  }
                  frame True {
                  }
                }
              }
              frame Enabled {
              }
            }
            n119 = Not(x="ReleaseTable") -> (.not. x?=w199:bool)
          }
          event "B_Stop": Value Change {
            n120 = event-data() -> ()  [unwired: 1 in, 6 out]
          }
          event "B_Disconnect": Value Change {
            n121 = event-data() -> ()  [unwired: 1 in, 6 out]
            n122 = Unbundle By Name(w213) -> ("conParam.type_con"=w217:enum16{"Serial", "TCP"})
            n123 = case shown="\"TCP\"" w217 {
              tunnel: w213 -> [w219 w223]
              tunnel: [w219 w221] -> w212
              tunnel: [w218 _] -> w214
              frame "Serial", Default {
                n124 = Unbundle By Name(w219) -> ("conParam.VISA"=w220:refnum<visa-resource-name>)
                n125 = VISA Close(VISA resource name=w220) -> (error out=w218:errorcluster)  [unwired: 1 in]
              }
              frame "TCP" {
                n126 = Unbundle By Name(w223) -> ("conParam.connection ID"=w224:refnum<k5>)
                n127 = TCP Close Connection(connection ID=w224) -> (connection ID out=w222:refnum<k5>)  [unwired: 2 in, 1 out]
                n128 = Bundle By Name(cluster=w223, "conParam.connection ID"=w222) -> (w221:T4)
              }
            }
            n129 = Not(x="B_Disconnect") -> (.not. x?=w215:bool)
          }
        }
        "error out" <- w19
        n130 = Unbundle By Name(w19) -> ("status"=w18:bool)
        n131 = Or(x=w18, y=w17) -> (x .or. y?=w16:bool)
      }
    }
  }
